vi "Video Toolset v10.0.0.vi"(9 "Capture Folder":path, 10 "Source Name":string, 11 "Autorun":bool) -> ()   [LabVIEW 2010]
uses:
  System.Windows.Forms
  drivers/DirectShow SDK/v10/DirectShow SDK.llb/DirectShow - Media State.ctl
  D:/Projekte/Promotion/Scripts/LabView/drivers/DirectShow SDK/lib/DirectShowLib-2005.dll
  drivers/DirectShow SDK/lib/DirectShowLib-2005.dll
  drivers/DirectShow SDK/v10/DirectShow SDK.llb/DirectShow - Capture Device.ctl
  drivers/DirectShow SDK/v10/DirectShow SDK.llb/DirectShow - Media Mode.ctl
  System.Drawing
  subvi/Remote Snapshot.vi
panel:
  in  "Autoclose":bool
  in  "Preview":refnum<k24>(container)
  in  "AutocloseText":string
  in  "AutorunText":string
  in  "Selector":u16(ring) items=["MJPG 1280x720, 30.00fps, 24bit", "MJPG 320x180, 30.00fps, 24bit", "MJPG 320x240, 30.00fps, 24bit", "MJPG 352x288, 30.00fps, 24bit", "MJPG 424x240, 30.00fps, 24bit", "MJPG 640x360, 30.00fps, 24bit", "MJPG 640x480, 30.00fps, 24bit", "MJPG 848x480, 30.00fps, 24bit", "MJPG 960x540, 30.00fps, 24bit", "YUY2 640x480, 30.00fps, 16bit", "YUY2 320x180, 30.00fps, 16bit", "YUY2 320x240, 30.00fps, 16bit", "YUY2 352x288, 30.00fps, 16bit", "YUY2 424x240, 30.00fps, 16bit", "YUY2 640x360, 30.00fps, 16bit", "YUY2 848x480, 20.00fps, 16bit", "YUY2 960x540, 15.00fps, 16bit", "YUY2 1280x720, 10.00fps, 16bit", "RGB 640x480, 30.00fps, 24bit", "RGB 320x180, 30.00fps, 24bit", "RGB 320x240, 30.00fps, 24bit", "RGB 352x288, 30.00fps, 24bit", "RGB 424x240, 30.00fps, 24bit", "RGB 640x360, 30.00fps, 24bit", "RGB 848x480, 20.00fps, 24bit", "RGB 960x540, 15.00fps, 24bit", "RGB 1280x720, 10.00fps, 24bit"]
  in  "WindowSnap":refnum<k24>(container)
  out "SnapSummary":string
  in  "Grab Window Image":bool
  in  "Pause":bool
  in  "Run":bool
  in  "Stop":bool
  in  "Capture":bool
  out "Summary":string
  in  "Grab Frame":bool
  in  "FrameGrab":refnum<k24>(container)
  out "Info":string
  in  "Fit Window":bool
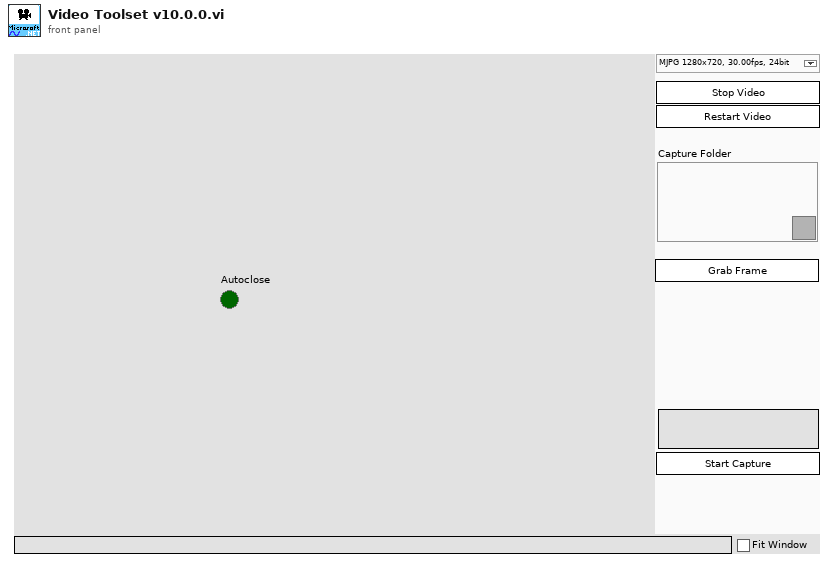
[diagram p1: front panel]
types:
  T1 = typedef "DirectShow - Media State.ctl" = enum16{"Stopped", "Playing", "Paused", "Recording"}
  T2 = typedef "DirectShow - Media Mode.ctl" = enum16{"Stop", "Run", "Pause"}
  T3 = typedef "DirectShow - Capture Device.ctl" = cluster{"DSDevice":refnum<k24>, "DevicePath":string, "Mon":refnum<k24>, "Name":string}
  T4 = enum8{"Enabled", "Disabled", "Disabled and Grayed Out"}
  T5 = enum16{"AnalogVideoIn", "Capture", "CC", "EDS", "NABTS", "Preview", "Still", "TeleText", "TimeCode", "VBI", "VideoPort", "VideoPortVBI"}
  T6 = cluster{"This VI":refnum<vi>, "Pane":refnum<vi>, "Timeout":i32, "Error":errorcluster, "Preview":refnum<k24>, "FrameGrab":refnum<k24>, "WindowSnap":refnum<k24>, "Video":T3, "Audio":T3, "VideoC":T3, "AudioC":T3, "Preview?":bool, "Capture?":bool, "ScaleWindow?":bool, "FrameGrabber?":bool, "IFilterGraph2":refnum<k24>, "ICaptureGraphBuilder2":refnum<k24>, "Video Caps":string[], "Audio Caps":string[], "CurrentVideo":string, "CurrentAudio":string, "MediaState":T1}
  T7 = typedef "sizeaction.ctl" = enum32{"Minimized", "Maximized", "Resized"}
  T8 = typedef "LVRectTypeDef.ctl" = cluster{"left":i16, "top":i16, "right":i16, "bottom":i16}
  T9 = cluster{"ID +Items":string[], "Items dup":string[], "Name":string}
  T10 = cluster{"ID +Items":string[], "Items dup":string[], "Name":string}[]
  T11 = typedef "imagedata.ctl" = cluster{"image type":i32, "image depth":i32, "image":u8[], "mask":u8[], "colors":u32[], "Rectangle":cluster{"left":i16, "top":i16, "right":i16, "bottom":i16}}
  T12 = enum32{"invalid app kind", "Development System", "Run Time System", "Student Edition", "Embedded LabVIEW", "Evaluation", "Custom"}
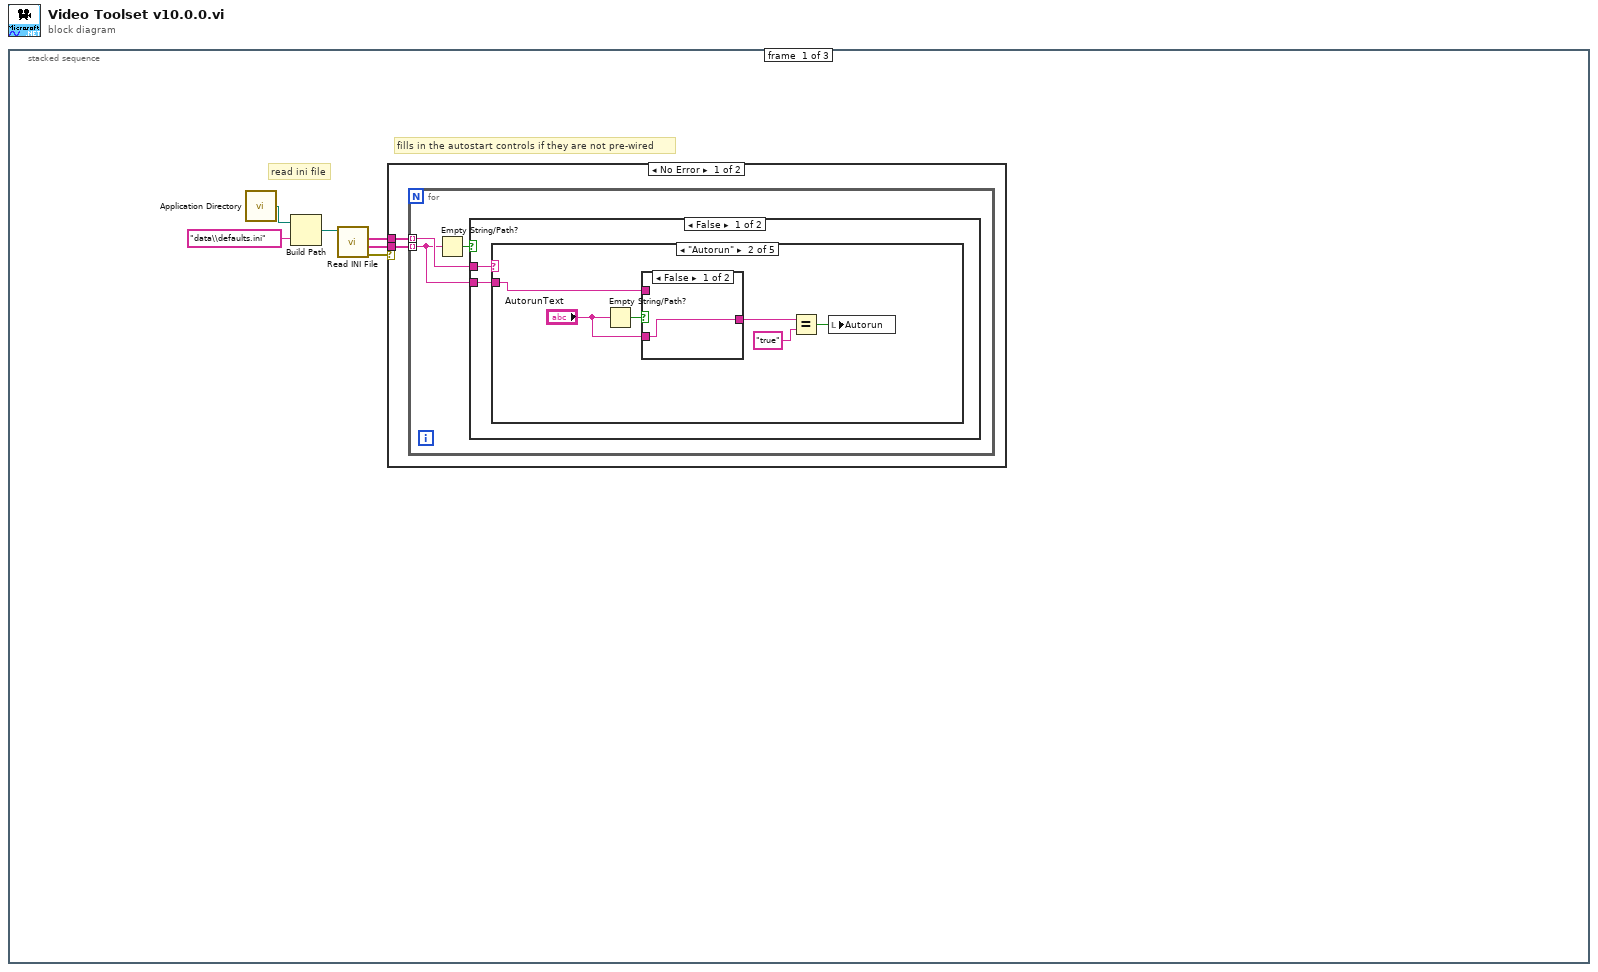
[diagram p0: block diagram]
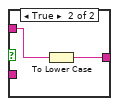
[diagram p3: hidden frame]
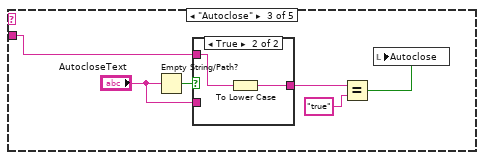
[diagram p4: hidden frame]
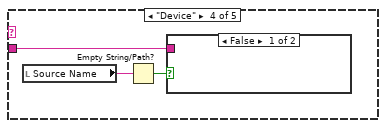
[diagram p6: hidden frame]
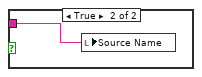
[diagram p7: hidden frame]
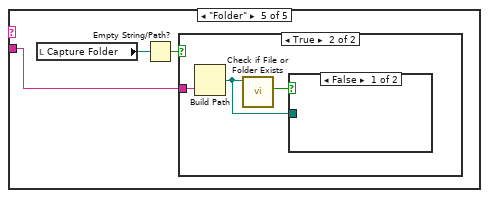
[diagram p8: hidden frame]
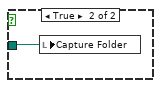
[diagram p10: hidden frame]
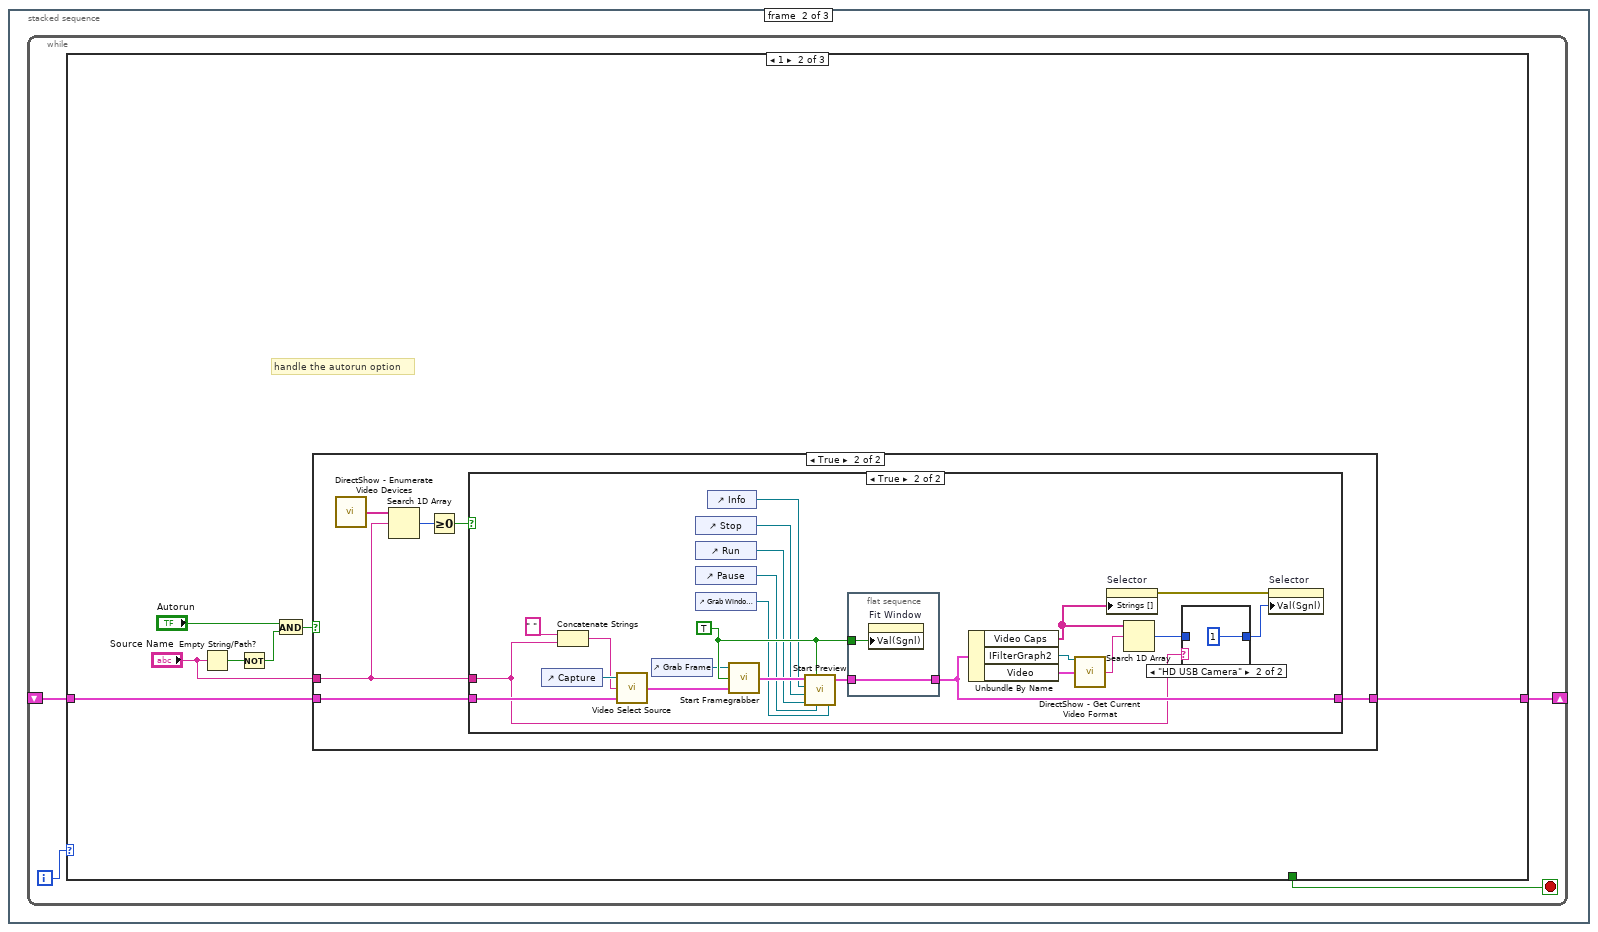
[diagram p13: hidden frame]
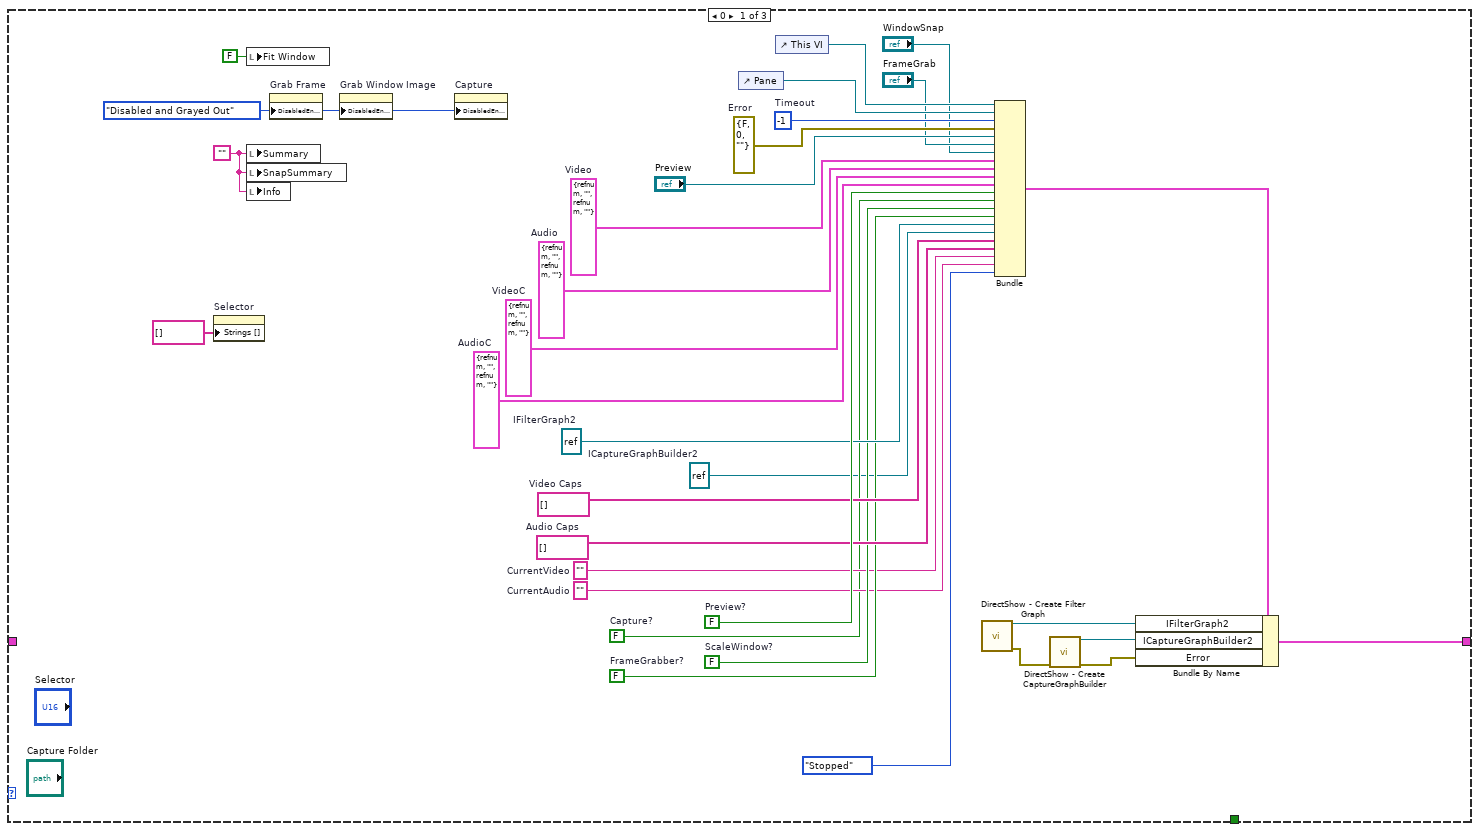
[diagram p14: hidden frame]
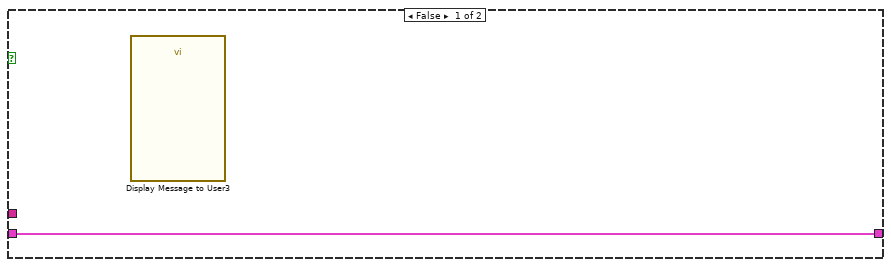
[diagram p16: hidden frame]
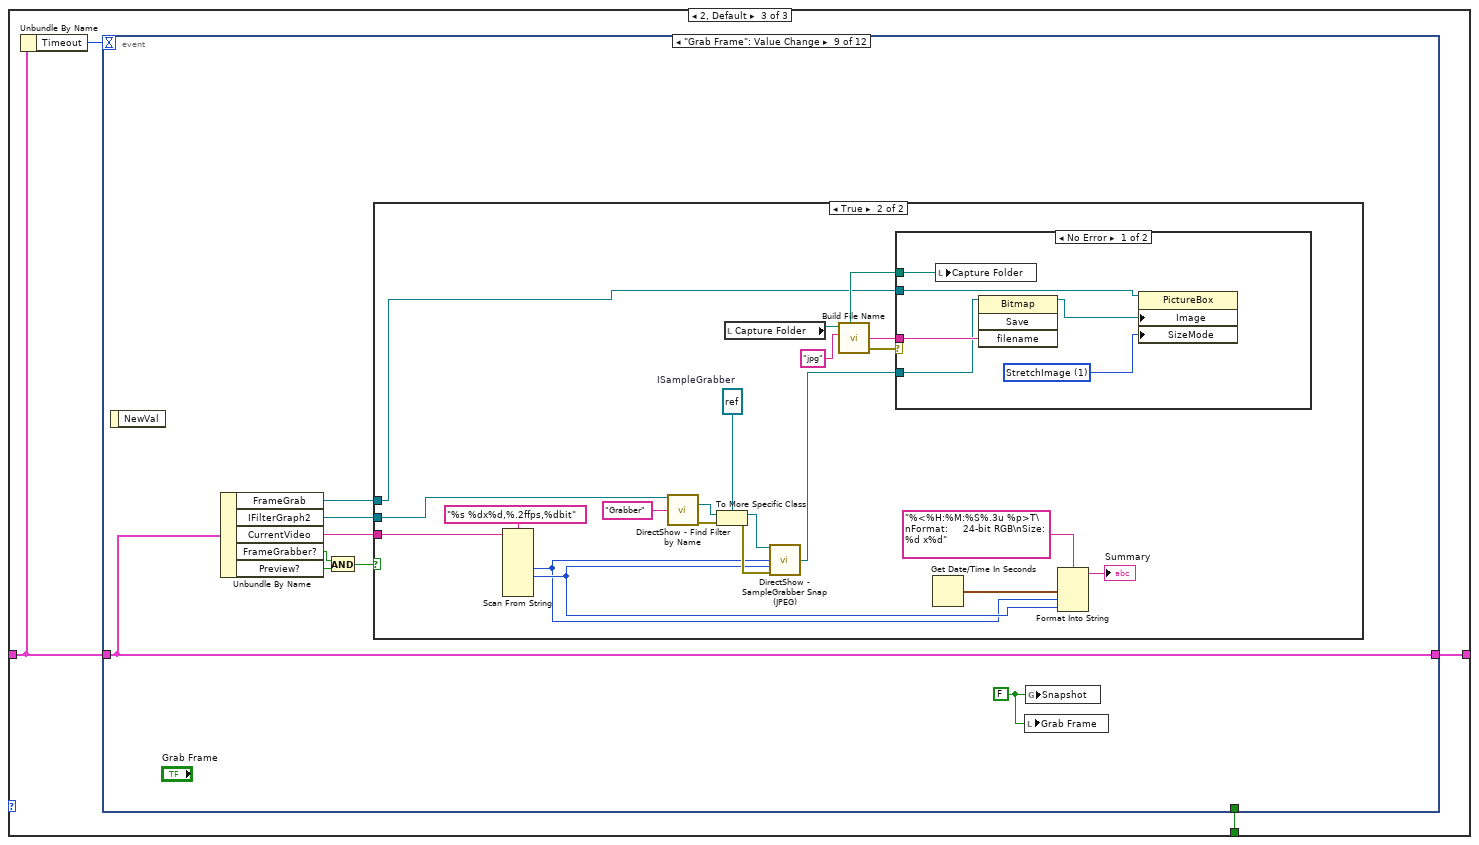
[diagram p18: hidden frame]
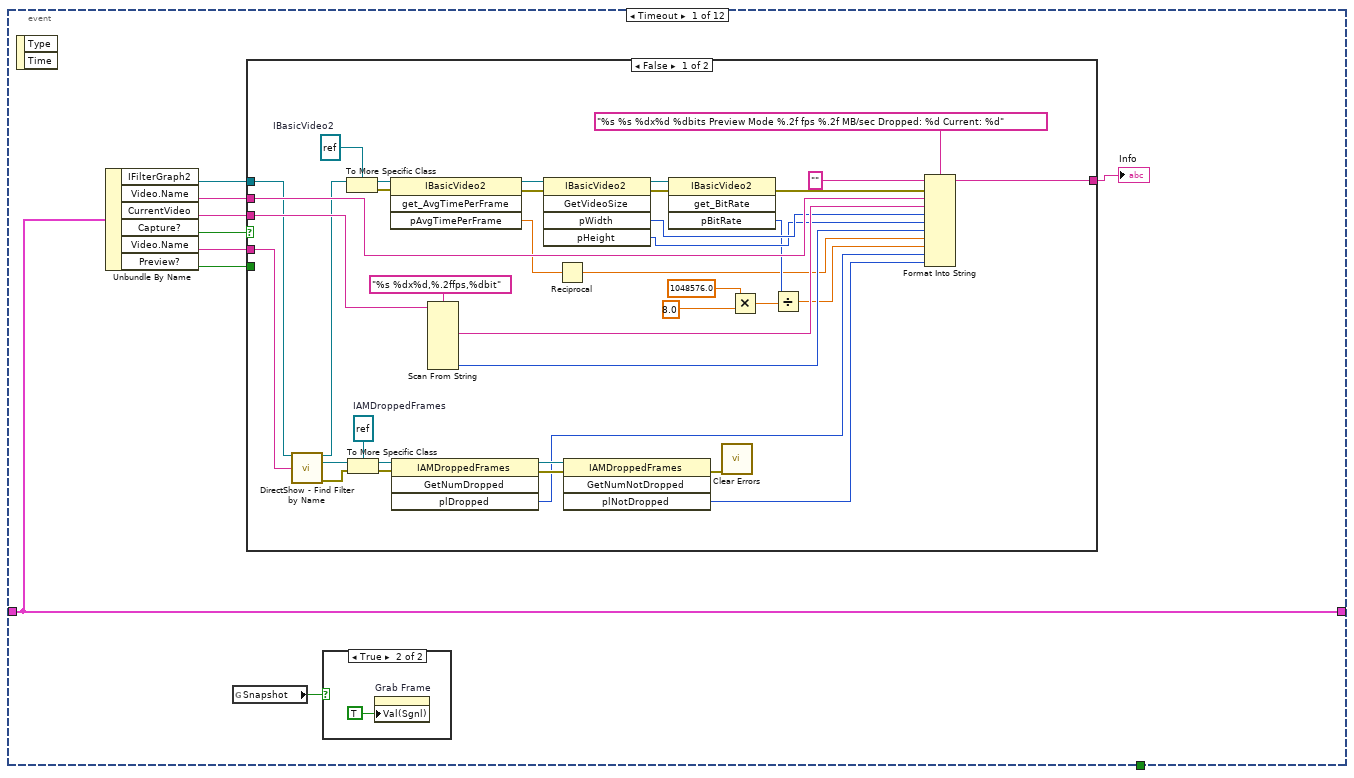
[diagram p19: hidden frame]
diagram:
  n1 = stacked-sequence {
    frame #0 {
      # "fills in the autostart controls if they are not pre-wired"
      # "read ini file"
      n2 = call <vilib>:"Application Directory.vi"() -> ("Application Directory"=w1:path)
      n3 = Build Path(base path=w1, name or relative path="data\\defaults.ini") -> (appended path=w5:path)
      n4 = call "Read INI File.vi"("configuration file path"=w5) -> ("error out"=w4:errorcluster, "values"=w2:string[], "keys"=w3:string[])  [unwired: 7 in, 1 out]
      n5 = case shown="No Error" w4 {
        tunnel: w3 -> [w8 _]
        tunnel: w2 -> [w7 _]
        frame No Error {
          n6 = for {
            tunnel: w8 -> [w10] mode=indexing
            tunnel: w7 -> [w9] mode=indexing
            n7 = Empty String/Path?(string/path=w9) -> (empty?=w11:bool)
            n8 = case shown="False" w11 {
              tunnel: w10 -> [w13 _]
              tunnel: w9 -> [w12 _]
              frame False {
                n9 = case shown="\"Autorun\"" w13 {
                  tunnel: w12 -> [_ w19 w23 w34 w38]
                  frame Default {
                  }
                  frame "Autorun" {
                    n10 = Empty String/Path?(string/path="AutorunText") -> (empty?=w17:bool)
                    n11 = case shown="False" w17 {
                      tunnel: w19 -> [_ w22]
                      tunnel: [w20 w21] -> w16
                      tunnel: "AutorunText" -> [w20 _]
                      frame False {
                      }
                      frame True {
                        n12 = To Lower Case(string=w22) -> (all lower case string=w21:string)
                      }
                    }
                    n13 = Equal?(x=w16, y="true") -> (x = y?=w14:bool)
                    n14 = local write "Autorun"(w14) -> ()
                  }
                  frame "Autoclose" {
                    n15 = Empty String/Path?(string/path="AutocloseText") -> (empty?=w24:bool)
                    n16 = case shown="True" w24 {
                      tunnel: [w29 w31] -> w27
                      tunnel: "AutocloseText" -> [w29 _]
                      tunnel: w23 -> [_ w30]
                      frame False {
                      }
                      frame True {
                        n17 = To Lower Case(string=w30) -> (all lower case string=w31:string)
                      }
                    }
                    n18 = Equal?(x=w27, y="true") -> (x = y?=w26:bool)
                    n19 = local write "Autoclose"(w26) -> ()
                  }
                  frame "Device" {
                    n20 = local read "Source Name"() -> (w33:string)
                    n21 = Empty String/Path?(string/path=w33) -> (empty?=w32:bool)
                    n22 = case shown="False" w32 {
                      tunnel: w34 -> [_ w35]
                      frame False {
                      }
                      frame True {
                        n23 = local write "Source Name"(w35) -> ()
                      }
                    }
                  }
                  frame "Folder" {
                    n24 = local read "Capture Folder"() -> (w37:path)
                    n25 = Empty String/Path?(string/path=w37) -> (empty?=w36:bool)
                    n26 = case shown="True" w36 {
                      tunnel: w38 -> [_ w41]
                      frame False {
                      }
                      frame True {
                        n27 = Build Path(name or relative path=w41) -> (appended path=w39:path)  [unwired: 1 in]
                        n28 = call <vilib>:"Check if File or Folder Exists.vi"("path"=w39) -> ("file or folder exists?"=w40:bool)  [unwired: 8 in, 2 out]
                        n29 = case shown="False" w40 {
                          tunnel: w39 -> [_ w42]
                          frame False {
                          }
                          frame True {
                            n30 = local write "Capture Folder"(w42) -> ()
                          }
                        }
                      }
                    }
                  }
                }
              }
              frame True {
              }
            }
          }
        }
        frame Error {
        }
      }
    }
    frame #1 {
      n31 = while {
        shift-right: [w45] -> _
        shift-left: _ -> [w44]
        i -> [w46]
        stop <- w43 stop-if-true
        n32 = case shown="1" w46 {
          tunnel: [w62 w81 w124] -> w45
          tunnel: w44 -> [_ w85 w123]
          tunnel: [_ _ w121] -> w43
          frame 0 {
            w47 = ""
            w55 = refnum<k24> refnum  # ICaptureGraphBuilder2
            w56 = FALSE  # Capture?
            w49 = T4."Disabled and Grayed Out" ("Disabled")
            w59 = ""  # CurrentAudio
            w60 = ""  # CurrentVideo
            w63 = FALSE  # FrameGrabber?
            w65 = FALSE  # ScaleWindow?
            w66 = string[] []  # Audio Caps
            w67 = string[] []  # Video Caps
            w70 = refnum<k24> refnum  # IFilterGraph2
            w71 = FALSE  # Preview?
            w72 = T3 {"DSDevice"=refnum, "DevicePath"="", "Mon"=refnum, "Name"=""}  # AudioC
            w73 = T3 {"DSDevice"=refnum, "DevicePath"="", "Mon"=refnum, "Name"=""}  # VideoC
            w74 = T3 {"DSDevice"=refnum, "DevicePath"="", "Mon"=refnum, "Name"=""}  # Audio
            w75 = T3 {"DSDevice"=refnum, "DevicePath"="", "Mon"=refnum, "Name"=""}  # Video
            w77 = errorcluster {"status"=FALSE, "code"=0, "source"=""}  # Error
            w78 = -1  # Timeout
            n33 = property on="Selector" class="Ring (strict)"("Strings []"=string[] []) -> ()  [unwired: 2 in, 2 out]
            n34 = local write "Fit Window"(FALSE ("Fit Window")) -> ()
            n35 = local write "Summary"(w47) -> ()
            n36 = local write "SnapSummary"(w47) -> ()
            n37 = local write "Info"(w47) -> ()
            n38 = property on="Grab Frame" class="Bool (strict)"("DisabledEnum"=w49) -> ()  [unwired: 2 in, 2 out]
            n39 = property on="Grab Window Image" class="Bool"("DisabledEnum"=w49) -> ()  [unwired: 2 in, 2 out]
            n40 = property on="Capture" class="Bool (strict)"("DisabledEnum"=w49) -> ()  [unwired: 2 in, 2 out]
            n41 = control-ref of="Pane"() -> (w58:refnum<vi>)
            n42 = control-ref of="This VI"() -> (w64:refnum<vi>)
            n43 = call "DirectShow - Create Filter Graph.vi"() -> ("IFilterGraph2"=w61:refnum<k24>, "error out"=w53:errorcluster)  [unwired: 14 in]
            n44 = Bundle("This VI"=w64, "Pane"=w58, "Timeout"=w78, "Error"=w77, "Preview"="Preview", "FrameGrab"="FrameGrab", "WindowSnap"="WindowSnap", "Video"=w75, "Audio"=w74, "VideoC"=w73, "AudioC"=w72, "Preview?"=w71, "Capture?"=w56, "ScaleWindow?"=w65, "FrameGrabber?"=w63, "IFilterGraph2"=w70, "ICaptureGraphBuilder2"=w55, "Video Caps"=w67, "Audio Caps"=w66, "CurrentVideo"=w60, "CurrentAudio"=w59, "MediaState"=DirectShow_-_Media_State."Stopped") -> (w68:T6)  [unwired: 1 in]
            n45 = call "DirectShow - Create CaptureGraphBuilder.vi"("error in (no error)"=w53) -> ("ICaptureGraphBuilder2"=w54:refnum<k24>, "error out"=w52:errorcluster)  [unwired: 13 in]
            n46 = Bundle By Name(cluster=w68, "IFilterGraph2"=w61, "ICaptureGraphBuilder2"=w54, "Error"=w52) -> (w62:T6)
          }
          frame 1 {
            # "handle the autorun option"
            n47 = Empty String/Path?(string/path="Source Name") -> (empty?=w80:bool)
            n48 = Not(x=w80) -> (.not. x?=w79:bool)
            n49 = And(x="Autorun", y=w79) -> (x .and. y?=w82:bool)
            n50 = case shown="True" w82 {
              tunnel: w85 -> [w86 w92]
              tunnel: "Source Name" -> [_ w90]
              tunnel: [w86 w91] -> w81
              frame False {
              }
              frame True {
                n51 = call "DirectShow - Enumerate Video Devices.vi"() -> ("Names"=w89:string[])  [unwired: 13 in, 2 out]
                n52 = Search 1D Array(1D array=w89, element=w90) -> (index of element=w88:i32)  [unwired: 1 in]
                n53 = Greater Or Equal To 0?(x=w88) -> (x >= 0?=w87:bool)
                n54 = case shown="True" w87 {
                  tunnel: w92 -> [w93 w115]
                  tunnel: [w93 w101] -> w91
                  tunnel: w90 -> [_ w97]
                  frame False {
                    n55 = call "Display Message to User3"() -> ()  [unwired: 10 in, 2 out]
                  }
                  frame True {
                    w116 = TRUE ("Value (Signaling)")
                    n56 = control-ref of="Capture"() -> (w112:refnum<vi>)
                    n57 = Concatenate Strings(" " ("string"), w97) -> (w104:string)
                    n58 = call "Video Select Source.vi"("Cluster In"=w115, "Source Name"=w104, "Bool Refnum"=w112) -> ("Cluster Out"=w114:T6)
                    n59 = control-ref of="Grab Frame"() -> (w111:refnum<vi>)
                    n60 = control-ref of="Stop"() -> (w106:refnum<vi>)
                    n61 = control-ref of="Run"() -> (w108:refnum<vi>)
                    n62 = control-ref of="Pause"() -> (w109:refnum<vi>)
                    n63 = control-ref of="Grab Window Image"() -> (w110:refnum<vi>)
                    n64 = control-ref of="Info"() -> (w107:refnum<vi>)
                    n65 = call "Start Framegrabber.vi"("Cluster In"=w114, "Enable?"=w116, "Bool Refnum"=w111) -> ("Cluster Out"=w113:T6)
                    n66 = call "Start Preview.vi"("Cluster In"=w113, "Start?"=w116, "Info"=w107, "Stop"=w106, "Pause"=w109, "Run"=w108, "Grab Window Image"=w110) -> ("Cluster Out"=w103:T6)  [unwired: 1 in]
                    n67 = flat-sequence {
                      tunnel: w116 -> [w120]
                      tunnel: [w119] -> w101
                      tunnel: w103 -> [w119]
                      frame #0 {
                        n68 = property on="Fit Window" class="Bool (strict)"("Val(Sgnl)"=w120) -> ()  [unwired: 2 in, 2 out]
                      }
                    }
                    n69 = Unbundle By Name(w101) -> ("Video Caps"=w102:string[], "IFilterGraph2"=w98:refnum<k24>, "Video"=w99:T3)
                    n70 = call "DirectShow - Get Current Video Format.vi"("IFilterGraph2"=w98, "Video"=w99) -> ("Abbreviated"=w100:string)  [unwired: 10 in, 3 out]
                    n71 = property on="Selector" class="Ring (strict)"("Strings []"=w102) -> (error out=w96:errorcluster)  [unwired: 2 in, 1 out]
                    n72 = Search 1D Array(1D array=w102, element=w100) -> (index of element=w94:i32)  [unwired: 1 in]
                    n73 = case shown="\"HD USB Camera\"" w97 {
                      tunnel: [w117 u16 1 ("Value (Signaling)")] -> w95
                      tunnel: w94 -> [w117 _]
                      frame "False", Default {
                      }
                      frame "HD USB Camera" {
                      }
                    }
                    n74 = property on="Selector" class="Ring (strict)"(error in=w96, "Val(Sgnl)"=w95) -> ()  [unwired: 1 in, 2 out]
                  }
                }
              }
            }
          }
          frame 2, Default {
            n75 = Unbundle By Name(w123) -> ("Timeout"=w122:i32)
            n76 = event shown="[8] \"Grab Frame\": Value Change" {
              selector: _ -> [_ _ _ _ _ _ _ _ _ _ _ _]
              dyn-events: _ -> [_ _ _ _ _ _ _ _ _ _ _ _]
              timeout: w122 -> [_ _ _ _ _ _ _ _ _ _ _ _]
              tunnel: [w133 w204 w226 w285 w395 w999 w1078 w1102 w1126 w1160 w1183 w1318] -> w124
              tunnel: w123 -> [w133 w204 w227 w306 w394 w1000 w1077 w1101 w1126 w1160 w1182 w1318]
              tunnel: [_ w208 _ _ w393 _ _ _ _ _ _ _] -> w121
              event Timeout {
                n77 = event-data() -> ()  [unwired: 1 in, 2 out]
                n78 = Unbundle By Name(w133) -> ("IFilterGraph2"=w132:refnum<k24>, "Video.Name"=w130:string, "CurrentVideo"=w131:string, "Capture?"=w129:bool, "Video.Name"=w127:string, "Preview?"=w126:bool)
                n79 = global read "Remote Snapshot.vi" "Snapshot"() -> (w125:bool)
                n80 = case shown="False" w129 {
                  tunnel: w132 -> [w144 w187]
                  tunnel: w131 -> [w162 w182]
                  tunnel: w130 -> [w160 w184]
                  tunnel: [w150 w185] -> w128
                  tunnel: w127 -> [w145 w188]
                  tunnel: w126 -> [_ _]
                  frame False {
                    w149 = refnum<k24> refnum  # IAMDroppedFrames
                    w172 = refnum<k24> refnum  # IBasicVideo2
                    n81 = call "DirectShow - Find Filter by Name.vi"("IFilterGraph2"=w144, "pName"=w145) -> ("IFilterGraph2 dup"=w143:refnum<k24>, "ppFilter"=w148:refnum<k24>, "error out"=w142:errorcluster)  [unwired: 11 in]
                    n82 = To More Specific Class(target class=w172, reference=w143) -> (specific class reference=w171:refnum<k24>, error out=w170:errorcluster)  [unwired: 1 in]
                    n83 = To More Specific Class(target class=w149, reference=w148, error in=w142) -> (specific class reference=w139:refnum<k24>, error out=w138:errorcluster)
                    n84 = invoke class="IBasicVideo2" method="get_AvgTimePerFrame"(reference=w171, error in=w170) -> (reference out=w169:refnum<k24>, error out=w168:errorcluster, "pAvgTimePerFrame"=w152:dbl)  [unwired: 2 in, 1 out]
                    n85 = invoke class="IAMDroppedFrames" method="GetNumDropped"(reference=w139, error in=w138) -> (reference out=w147:refnum<k24>, error out=w146:errorcluster, "plDropped"=w137:i32)  [unwired: 2 in, 1 out]
                    n86 = Scan From String(format string="%s %dx%d,%.2ffps,%dbit", input string=w162) -> (output 1=w159:string, output 5=w158:i32)  [unwired: 10 in, 3 out]
                    n87 = invoke class="IBasicVideo2" method="GetVideoSize"(reference=w169, error in=w168) -> (reference out=w167:refnum<k24>, error out=w166:errorcluster, "pWidth"=w157:i32, "pHeight"=w156:i32)  [unwired: 3 in, 1 out]
                    n88 = Reciprocal(x=w152) -> (1/x=w151:dbl)
                    n89 = invoke class="IAMDroppedFrames" method="GetNumNotDropped"(reference=w147, error in=w146) -> (error out=w135:errorcluster, "plNotDropped"=w136:i32)  [unwired: 2 in, 2 out]
                    n90 = invoke class="IBasicVideo2" method="get_BitRate"(reference=w167, error in=w166) -> (error out=w165:errorcluster, "pBitRate"=w155:i32)  [unwired: 2 in, 2 out]
                    n91 = call <vilib>:"Clear Errors.vi"("error in (no error)"=w135) -> ()  [unwired: 6 in, 1 out]
                    n92 = Multiply(x=1048576.0, y=8.0) -> (x*y=w141:dbl)
                    n93 = Divide(x=w155, y=w141) -> (x/y=w153:dbl)
                    n94 = Format Into String(format string="%s %s %dx%d %dbits Preview Mode %.2f fps %.2f MB/sec Dropped: %d Current: %d", initial string="", error in=w165, w160, w159, w157, w156, w158, w151, w153, w137, w136) -> (resulting string=w150:string)  [unwired: 1 out]
                  }
                  frame True {
                    w192 = refnum<k24> refnum  # IAMDroppedFrames
                    n95 = call "DirectShow - Find Filter by Name.vi"("IFilterGraph2"=w187, "pName"=w188) -> ("ppFilter"=w191:refnum<k24>, "error out"=w190:errorcluster)  [unwired: 11 in, 1 out]
                    n96 = To More Specific Class(target class=w192, reference=w191, error in=w190) -> (specific class reference=w173:refnum<k24>, error out=w189:errorcluster)
                    n97 = Scan From String(format string="%s %dx%d,%.2ffps,%dbit", input string=w182) -> (output 1=w181:string, output 2=w180:i32, output 3=w179:i32, output 4=w177:dbl, output 5=w178:i32)  [unwired: 7 in, 3 out]
                    n98 = Not A Number/Path/Refnum?(number/path/refnum=w173) -> (NaN/Path/Refnum?=w174:bool)
                    n99 = case shown="False" w174 {
                      tunnel: w173 -> [w196 _]
                      tunnel: w189 -> [w195 _]
                      tunnel: [w194 w199] -> w176
                      tunnel: [w193 w199] -> w175
                      frame False {
                        n100 = invoke class="IAMDroppedFrames" method="GetNumDropped"(reference=w196, error in=w195) -> (reference out=w198:refnum<k24>, error out=w197:errorcluster, "plDropped"=w194:i32)  [unwired: 2 in, 1 out]
                        n101 = invoke class="IAMDroppedFrames" method="GetNumNotDropped"(reference=w198, error in=w197) -> ("plNotDropped"=w193:i32)  [unwired: 2 in, 3 out]
                      }
                      frame True {
                        w199 = 0 ("plDropped")
                      }
                    }
                    n102 = Format Into String(format string="%s %s %dx%d %dbits Capture Mode %.2f fps Dropped: %d Current: %d", w184, w181, w180, w179, w178, w177, w176, w175) -> (resulting string=w185:string)  [unwired: 2 in, 1 out]
                  }
                }
                "Info" <- w128
                n103 = case shown="True" w125 {
                  frame False {
                  }
                  frame True {
                    n104 = property on="Grab Frame" class="Bool (strict)"("Val(Sgnl)"=TRUE) -> ()  [unwired: 2 in, 2 out]
                  }
                }
              }
              event Panel Close? {
                w208 = TRUE ("Discard?")
                n105 = event-data() -> ()  [unwired: 1 in, 3 out]
                n106 = Unbundle By Name(w204) -> ("ICaptureGraphBuilder2"=w200:refnum<k24>, "Capture?"=w201:bool, "IFilterGraph2"=w207:refnum<k24>, "Error"=w206:errorcluster, "Preview?"=w205:bool)
                n107 = case shown="True" w205 {
                  tunnel: w207 -> [w210 w218]
                  tunnel: w206 -> [w209 _]
                  tunnel: [w210 w213] -> w203
                  tunnel: [w209 w211] -> w202
                  tunnel: w201 -> [_ w216]
                  tunnel: w200 -> [_ w215]
                  frame False {
                  }
                  frame True {
                    n108 = call "DirectShow - Media Control - StartStopPause.vi"("IFilterGraph2"=w218, "Mode"=DirectShow_-_Media_Mode."Stop") -> ("IFilterGraph2 dup"=w212:refnum<k24>, "error out"=w214:errorcluster)  [unwired: 12 in]
                    n109 = case shown="True" w216 {
                      tunnel: w215 -> [_ w224]
                      tunnel: w214 -> [w219 w223]
                      tunnel: [w220 w222] -> w213
                      tunnel: w212 -> [w220 w222]
                      tunnel: [w219 w221] -> w211
                      frame False {
                      }
                      frame True {
                        n110 = call "DirectShow - Release Object.vi"("o"=w224, "error in (no error)"=w223) -> ("error out"=w221:errorcluster)  [unwired: 13 in]
                      }
                    }
                  }
                }
                n111 = call "DirectShow - Release Object.vi"("o"=w203, "error in (no error)"=w202) -> ()  [unwired: 13 in, 1 out]
                n112 = event-data("Discard?"=w208) -> ()  [unwired: 1 in, 1 out]
              }
              event Panel Resize {
                n113 = event-data() -> ("Act"=w225:T7)  [unwired: 1 in]
                n114 = case shown="\"Maximized\", Default" w225 {
                  tunnel: w227 -> [w228 w235]
                  tunnel: [w228 w234] -> w226
                  frame "Minimized" {
                  }
                  frame "Maximized", Default {
                    n115 = Unbundle By Name(w235) -> ("Pane"=w232:refnum<vi>, "Error"=w233:errorcluster, "IFilterGraph2"=w231:refnum<k24>, "ScaleWindow?"=w229:bool)
                    n116 = case shown="True" w229 {
                      tunnel: w233 -> [w236 w247]
                      tunnel: w232 -> [_ w246]
                      tunnel: w231 -> [_ w244]
                      tunnel: [w236 w240] -> w230
                      frame False {
                      }
                      frame True {
                        w239 = 0 ("left")
                        w245 = refnum<k24> refnum  # IVideoWindow
                        n117 = property class="Pane"(reference=w246, error in=w247) -> (error out=w243:errorcluster, "ContentBnds"=w252:T8)  [unwired: 1 out]
                        n118 = Unbundle(w252) -> ("left"=w248:i16, "top"=w250:i16, "right"=w249:i16, "bottom"=w251:i16)
                        n119 = Subtract(x=w249, y=w248) -> (x-y=w238:i16)
                        n120 = Subtract(x=w251, y=w250) -> (x-y=w237:i16)
                        n121 = To More Specific Class(target class=w245, reference=w244, error in=w243) -> (specific class reference=w242:refnum<k24>, error out=w241:errorcluster)
                        n122 = invoke class="IVideoWindow" method="SetWindowPosition"(reference=w242, error in=w241, "left"=w239, "top"=w239, "width"=w238, "height"=w237) -> (error out=w240:errorcluster)  [unwired: 1 in, 6 out]
                      }
                    }
                    n123 = Bundle By Name(cluster=w235, "Error"=w230) -> (w234:T6)
                  }
                }
              }
              event Menu Activation? {
                w271 = "(none)" ("Name")
                # "Disable Menu When in Capture Mode"
                n124 = event-data() -> ("MenuRef"=w257:refnum<k9>)  [unwired: 1 in]
                n125 = call "DirectShow - Enumerate Video Devices.vi"() -> ("Names"=w323:string[])  [unwired: 13 in, 2 out]
                n126 = call "DirectShow - Enumerate Audio Devices.vi"() -> ("Names"=w322:string[])  [unwired: 13 in, 2 out]
                n127 = call "DirectShow - Enumerate Video Compressors.vi"() -> ("Names"=w321:string[])  [unwired: 13 in, 2 out]
                n128 = call "DirectShow - Enumerate Audio Compressors.vi"() -> ("Names"=w320:string[])  [unwired: 13 in, 2 out]
                n129 = call "Logical String Array Sort.vi"("Unsorted List"=w323) -> ("Sorted List"=w298:string[])  [unwired: 18 in]
                n130 = call "Logical String Array Sort.vi"("Unsorted List"=w322) -> ("Sorted List"=w297:string[])  [unwired: 18 in]
                n131 = call "Logical String Array Sort.vi"("Unsorted List"=w321) -> ("Sorted List"=w296:string[])  [unwired: 18 in]
                n132 = call "Logical String Array Sort.vi"("Unsorted List"=w320) -> ("Sorted List"=w295:string[])  [unwired: 18 in]
                n133 = Build Array (concatenate)(w271, w298) -> (w277:string[])
                n134 = Build Array (concatenate)(w271, w297) -> (w273:string[])
                n135 = Build Array (concatenate)(w271, w296) -> (w270:string[])
                n136 = Build Array (concatenate)(w271, w295) -> (w269:string[])
                n137 = Unbundle By Name(w306) -> ("Capture?"=w258:bool, "Preview?"=w259:bool, "Video.Name"=w289:string, "Audio.Name"=w290:string, "VideoC.Name"=w309:string, "AudioC.Name"=w319:string)
                n138 = call "DirectShow - Menu - Append Item ID.vi"("ID"="Video:" ("tag"), "Items"=w277) -> ("ID +Items"=w274:string[], "Items dup"=w275:string[])  [unwired: 12 in]
                n139 = call "DirectShow - Menu - Append Item ID.vi"("ID"="VideoC:" ("tag"), "Items"=w270) -> ("ID +Items"=w265:string[], "Items dup"=w262:string[])  [unwired: 12 in]
                n140 = call "DirectShow - Menu - Append Item ID.vi"("ID"="Audio:" ("tag"), "Items"=w273) -> ("ID +Items"=w266:string[], "Items dup"=w263:string[])  [unwired: 12 in]
                n141 = call "DirectShow - Menu - Append Item ID.vi"("ID"="AudioC:" ("tag"), "Items"=w269) -> ("ID +Items"=w264:string[], "Items dup"=w261:string[])  [unwired: 12 in]
                n142 = Not(x=w258) -> (.not. x?=w253:bool)
                n143 = Bundle("ID +Items"=w274, "Items dup"=w275, "Name"=w289) -> (w328:T9)  [unwired: 1 in]
                n144 = Bundle("ID +Items"=w266, "Items dup"=w263, "Name"=w290) -> (w327:T9)  [unwired: 1 in]
                n145 = Bundle("ID +Items"=w265, "Items dup"=w262, "Name"=w309) -> (w326:T9)  [unwired: 1 in]
                n146 = Bundle("ID +Items"=w264, "Items dup"=w261, "Name"=w319) -> (w325:T9)  [unwired: 1 in]
                n147 = Build Array(w328, w327, w326, w325) -> (w324:T10)
                n148 = Not(x=w259) -> (.not. x?=w260:bool)
                n149 = for {
                  tunnel: w257 -> [w345]
                  tunnel: string[] ["Video Devices", "Audio Devices", "Video Compressors", "Audio Compressors"] -> [w344] mode=indexing
                  tunnel: w324 -> [w343] mode=indexing
                  tunnel: [w338] -> w318
                  tunnel: [w337] -> w317
                  tunnel: w260 -> [w336]
                  n150 = Unbundle(w343) -> ("ID +Items"=w341:string[], "Items dup"=w342:string[], "Name"=w339:string)
                  n151 = Empty String/Path?(string/path=w339) -> (empty?=w340:bool)
                  n152 = case shown="True" w340 {
                    tunnel: w345 -> [w359 w382]
                    tunnel: w344 -> [w351 w374]
                    tunnel: w342 -> [w348 w369]
                    tunnel: w341 -> [w347 w370]
                    tunnel: w339 -> [_ w373]
                    tunnel: [w350 w372] -> w338
                    tunnel: [w349 w371] -> w337
                    tunnel: w336 -> [w346 w368]
                    frame True {
                      n153 = Get Menu Item Info(7:w351, 11:w359) -> (0:w356:errorcluster, 3:w357:refnum<k9>, 5:w358:string[])  [unwired: 1 in, 4 out]
                      n154 = Delete Menu Items(6:w356, 7:w358, 8:w351, 9:w357) -> (0:w354:errorcluster, 3:w355:refnum<k9>)
                      n155 = Insert Menu Items(5:w351, 6:w354, 7:w347, 8:w348, 9:w355) -> (0:w353:errorcluster, 3:w352:refnum<k9>)  [unwired: 1 in, 1 out]
                      n156 = for {
                        shift-right: [w365] -> w350
                        shift-left: w352 -> [w366]
                        shift-right: [w364] -> w349
                        shift-left: w353 -> [w367]
                        tunnel: w347 -> [w363] mode=indexing
                        tunnel: w346 -> [w360]
                        i -> [w361]
                        n157 = Equal To 0?(x=w361) -> (x = 0?=w362:bool)
                        n158 = Set Menu Item Info(6:w362, 7:w363, 8:w367, 9:w360, 11:w366) -> (0:w364:errorcluster, 3:w365:refnum<k9>)  [unwired: 2 in]
                      }
                    }
                    frame False {
                      n159 = Get Menu Item Info(7:w374, 11:w382) -> (0:w379:errorcluster, 3:w380:refnum<k9>, 5:w381:string[])  [unwired: 1 in, 4 out]
                      n160 = Delete Menu Items(6:w379, 7:w381, 8:w374, 9:w380) -> (0:w377:errorcluster, 3:w378:refnum<k9>)
                      n161 = Insert Menu Items(5:w374, 6:w377, 7:w370, 8:w369, 9:w378) -> (0:w376:errorcluster, 3:w375:refnum<k9>)  [unwired: 1 in, 1 out]
                      n162 = for {
                        shift-right: [w389] -> w372
                        shift-left: w375 -> [w390]
                        shift-right: [w388] -> w371
                        shift-left: w376 -> [w391]
                        tunnel: w370 -> [w387] mode=indexing
                        tunnel: w373 -> [w385]
                        tunnel: w369 -> [w386] mode=indexing
                        tunnel: w368 -> [w383]
                        n163 = Equal?(x=w386, y=w385) -> (x = y?=w384:bool)
                        n164 = Set Menu Item Info(6:w384, 7:w387, 8:w391, 9:w383, 11:w390) -> (0:w388:errorcluster, 3:w389:refnum<k9>)  [unwired: 2 in]
                      }
                    }
                  }
                }
                n165 = Empty String/Path?(string/path=w289) -> (empty?=w313:bool)
                n166 = Empty String/Path?(string/path=w290) -> (empty?=w312:bool)
                n167 = Not(x=w313) -> (.not. x?=w256:bool)
                n168 = Not(x=w312) -> (.not. x?=w280:bool)
                n169 = Unbundle By Name(w306) -> ("Video Caps"=w303:string[], "Audio Caps"=w300:string[], "FrameGrabber?"=w291:bool, "IFilterGraph2"=w288:refnum<k24>, "Video"=w279:T3, "Audio"=w278:T3)
                n170 = Empty String/Path?(string/path=w309) -> (empty?=w307:bool)
                n171 = Not(x=w307) -> (.not. x?=w308:bool)
                n172 = Unbundle By Name(w306) -> ("Preview?"=w254:bool)
                n173 = And(x=w254, y=w280) -> (x .and. y?=w281:bool)
                n174 = And(x=w254, y=w256) -> (x .and. y?=w282:bool)
                n175 = Or(x=w256, y=w280) -> (x .or. y?=w310:bool)
                n176 = Build Array(w256, w280, w310, w256, w256, w308, w280, w256, w256, w256, w256, w280, w280, w280, w256, w280, w282, w281, w253, w253) -> (w311:bool[])
                n177 = for {
                  tunnel: w318 -> [w335]
                  tunnel: w317 -> [w334]
                  tunnel: string[] ["Video Compressors", "Audio Compressors", "Property Pages", "Video Capture Device", "Video Capture Pin", "Video Compressor", "Audio Capture Device", "Video Frame Format", "Video Frame Bits", "Video Frame Size", "Video Frame Rate", "Audio Channels", "Audio Sampling Rate", "Audio Sample Size", "Video Capabilities", "Audio Capabilities", "Video Renderer Stats", "Audio Renderer Stats", "Devices", "Options"] -> [w333] mode=indexing
                  tunnel: [w332] -> w315
                  tunnel: [w331] -> w314
                  tunnel: w311 -> [w330] mode=indexing
                  n178 = Set Menu Item Info(7:w333, 8:w334, 9:w330, 11:w335) -> (0:w331:errorcluster, 3:w332:refnum<k9>)  [unwired: 3 in]
                }
                n179 = call "DirectShow - Get Current Video Format.vi"("IFilterGraph2"=w288, "Video"=w279) -> ("IFIlterGraph2 dup"=w286:refnum<k24>, "Abbreviated"=w284:string, "error out"=w287:errorcluster)  [unwired: 10 in, 1 out]
                n180 = Set Menu Item Info(6:w254, 7:"Preview", 8:w314, 9:w256, 11:w315) -> (0:w304:errorcluster, 3:w305:refnum<k9>)  [unwired: 2 in]
                n181 = call "DirectShow - Get Current Audio Format.vi"("IFilterGraph2"=w286, "Audio"=w278, "error in (no error)"=w287) -> ("Abbreviated"=w283:string)  [unwired: 9 in, 3 out]
                n182 = call "DirectShow - Menu - Add Video Items.vi"("Menu"=w305, "Video Caps"=w303, "CurrentVideo"=w284, "error in (no error)"=w304) -> ("Menu out"=w302:refnum<k9>, "error out"=w301:errorcluster)  [unwired: 10 in]
                n183 = call "DirectShow - Menu - Add Audio Items.vi"("Menu"=w302, "Audio Caps"=w300, "CurrentAudio"=w283, "error in (no error)"=w301) -> ("Menu out"=w294:refnum<k9>, "error out"=w293:errorcluster)  [unwired: 10 in]
                n184 = Bundle By Name(cluster=w306, "CurrentVideo"=w284, "CurrentAudio"=w283) -> (w285:T6)
                n185 = Compound Arithmetic op=AND(w256, w253, invert w254) -> (w255:bool)
                n186 = Set Menu Item Info(6:w291, 7:"Enable Frame Grabber", 8:w293, 9:w255, 11:w294) -> ()  [unwired: 2 in, 2 out]
                n187 = event-data() -> ()  [unwired: 2 in, 1 out]
              }
              event Menu Selection (User) {
                n188 = event-data() -> ("MenuRef"=w392:refnum<k9>, "ItemTag"=w396:string)  [unwired: 1 in]
                n189 = case shown="\"Unknown\", Default" w396 {
                  selector: w396 -> [_ w431 w928 w935 _ _ _ _]
                  tunnel: [w399 w422 w919 w936 w945 w950 w972 w994] -> w395
                  tunnel: w394 -> [w399 w428 w920 w932 w945 w950 w972 w994]
                  tunnel: [TRUE _ _ _ _ _ _ _] -> w393
                  tunnel: w392 -> [_ _ w931 w940 _ _ _ _]
                  frame "Exit" {
                    n190 = Unbundle By Name(w399) -> ("ICaptureGraphBuilder2"=w398:refnum<k24>, "Capture?"=w397:bool, "IFilterGraph2"=w404:refnum<k24>, "Error"=w403:errorcluster, "Preview?"=w402:bool)
                    n191 = case shown="True" w402 {
                      tunnel: w404 -> [w407 w415]
                      tunnel: w403 -> [w406 _]
                      tunnel: [w407 w412] -> w401
                      tunnel: [w406 w411] -> w400
                      tunnel: w398 -> [_ w409]
                      tunnel: w397 -> [_ w408]
                      frame False {
                      }
                      frame True {
                        n192 = call "DirectShow - Media Control - StartStopPause.vi"("IFilterGraph2"=w415, "Mode"=DirectShow_-_Media_Mode."Stop") -> ("IFilterGraph2 dup"=w410:refnum<k24>, "error out"=w413:errorcluster)  [unwired: 12 in]
                        n193 = case shown="True" w408 {
                          tunnel: w409 -> [_ w421]
                          tunnel: w413 -> [w416 w420]
                          tunnel: [w417 w419] -> w412
                          tunnel: w410 -> [w417 w419]
                          tunnel: [w416 w418] -> w411
                          frame False {
                          }
                          frame True {
                            n194 = call "DirectShow - Release Object.vi"("o"=w421, "error in (no error)"=w420) -> ("error out"=w418:errorcluster)  [unwired: 13 in]
                          }
                        }
                      }
                    }
                    n195 = call "DirectShow - Release Object.vi"("o"=w401, "error in (no error)"=w400) -> ()  [unwired: 13 in, 1 out]
                  }
                  frame "Unknown", Default {
                    n196 = Search/Split String(string=w431, search string/char (-)=":") -> (substring before match=w429:string, match + rest of string=w427:string)  [unwired: 1 in, 1 out]
                    n197 = case shown="\"Video\"" w429 {
                      tunnel: [w432 w433 w451 w502 w532 w558 w568 w575 w582 w590 w660 w729 w799 w859 w882 w904] -> w422
                      tunnel: w428 -> [w432 w435 w443 w496 w525 w558 w568 w575 w582 w595 w664 w733 w803 w874 w895 w916]
                      tunnel: w427 -> [_ w436 w454 w505 w535 _ _ _ _ w596 w665 w734 w804 w875 w896 w917]
                      frame "Unknown", Default {
                      }
                      frame "Video" {
                        n198 = control-ref of="Capture"() -> (w434:refnum<vi>)
                        n199 = call "Video Select Source.vi"("Cluster In"=w435, "Source Name"=w436, "Bool Refnum"=w434) -> ("Cluster Out"=w433:T6)
                      }
                      frame "Audio" {
                        n200 = call "DirectShow - Enumerate Audio Devices.vi"() -> ("Devices"=w450:T3[], "Names"=w449:string[])  [unwired: 13 in, 1 out]
                        n201 = Search/Split String(string=w454, offset (0)=1) -> (match + rest of string=w452:string)  [unwired: 1 in, 2 out]
                        n202 = Search 1D Array(1D array=w449, element=w452) -> (index of element=w446:i32)  [unwired: 1 in]
                        n203 = Unbundle By Name(w443) -> ("IFilterGraph2"=w442:refnum<k24>, "Audio.Name"=w441:string)
                        n204 = Index Array(array=w450, index=w446) -> (element=w447:T3)
                        n205 = Less Than 0?(x=w446) -> (x < 0?=w445:bool)
                        n206 = Select(t=T3 {"DSDevice"=refnum, "DevicePath"="", "Mon"=refnum, "Name"=""}, s=w445, f=w447) -> (s? t:f=w438:T3)
                        n207 = case shown="False" w445 {
                          tunnel: w438 -> [w461 _]
                          tunnel: [w460 _] -> w444
                          tunnel: w442 -> [w459 w487]
                          tunnel: w441 -> [w457 w486]
                          tunnel: [w456 w484] -> w439
                          tunnel: [T4."Enabled" ("Disabled") T4."Disabled and Grayed Out" ("Disabled")] -> w437
                          frame False {
                            n208 = Empty String/Path?(string/path=w457) -> (empty?=w458:bool)
                            n209 = case shown="False" w458 {
                              tunnel: w461 -> [w467 w479]
                              tunnel: [w464 w476] -> w460
                              tunnel: w459 -> [w463 w473]
                              tunnel: w457 -> [_ w472]
                              tunnel: [w462 w471] -> w456
                              frame True {
                                n210 = call "DirectShow - Add Source Filter for Moniker.vi"("IFilterGraph2"=w463, "Device"=w467) -> ("IFilterGraph2 dup"=w462:refnum<k24>, "ppFilter"=w468:refnum<k24>, "error out"=w469:errorcluster)  [unwired: 11 in]
                                n211 = call "DirectShow - Find Pin ByCategory.vi"("Source"=w468, "Category"=T5."Capture", "error in (no error)"=w469) -> ("DS_Pin"=w465:refnum<k24>, "error out"=w466:errorcluster)  [unwired: 11 in]
                                n212 = call "DirectShow - Get Audio Stream Parameters.vi"("Stream"=w465, "error in (no error)"=w466) -> ("Abbreviated"=w464:string[])  [unwired: 9 in, 4 out]
                              }
                              frame False {
                                n213 = call "DirectShow - Delete Filter by Name.vi"("IFilterGraph2"=w473, "pName"=w472) -> ("IFilterGraph2 dup"=w475:refnum<k24>, "error out"=w474:errorcluster)  [unwired: 12 in]
                                n214 = call "DirectShow - Add Source Filter for Moniker.vi"("IFilterGraph2"=w475, "Device"=w479, "error in (no error)"=w474) -> ("IFilterGraph2 dup"=w471:refnum<k24>, "ppFilter"=w480:refnum<k24>, "error out"=w481:errorcluster)  [unwired: 10 in]
                                n215 = call "DirectShow - Find Pin ByCategory.vi"("Source"=w480, "Category"=T5."Capture", "error in (no error)"=w481) -> ("DS_Pin"=w477:refnum<k24>, "error out"=w478:errorcluster)  [unwired: 11 in]
                                n216 = call "DirectShow - Get Audio Stream Parameters.vi"("Stream"=w477, "error in (no error)"=w478) -> ("Abbreviated"=w476:string[])  [unwired: 9 in, 4 out]
                              }
                            }
                          }
                          frame True {
                            n217 = Empty String/Path?(string/path=w486) -> (empty?=w485:bool)
                            n218 = case shown="False" w485 {
                              tunnel: w487 -> [w490 w491]
                              tunnel: w486 -> [w489 _]
                              tunnel: [w488 w491] -> w484
                              frame False {
                                n219 = call "DirectShow - Delete Filter by Name.vi"("IFilterGraph2"=w490, "pName"=w489) -> ("IFilterGraph2 dup"=w488:refnum<k24>)  [unwired: 12 in, 1 out]
                              }
                              frame True {
                              }
                            }
                          }
                        }
                        n220 = call "DirectShow - Get Current Audio Format.vi"("IFilterGraph2"=w439, "Audio"=w438) -> ("Abbreviated"=w440:string)  [unwired: 10 in, 3 out]
                        n221 = property on="Capture" class="Bool (strict)"("DisabledEnum"=w437) -> ()  [unwired: 2 in, 2 out]
                        n222 = Bundle By Name(cluster=w443, "CurrentAudio"=w440, "Audio"=w438, "Audio Caps"=w444) -> (w451:T6)
                      }
                      frame "VideoC" {
                        n223 = call "DirectShow - Enumerate Video Compressors.vi"() -> ("Devices"=w501:T3[], "Names"=w500:string[])  [unwired: 13 in, 1 out]
                        n224 = Search/Split String(string=w505, offset (0)=1) -> (match + rest of string=w503:string)  [unwired: 1 in, 2 out]
                        n225 = Search 1D Array(1D array=w500, element=w503) -> (index of element=w498:i32)  [unwired: 1 in]
                        n226 = Unbundle By Name(w496) -> ("IFilterGraph2"=w495:refnum<k24>, "VideoC.Name"=w494:string)
                        n227 = Less Than 0?(x=w498) -> (x < 0?=w493:bool)
                        n228 = Index Array(array=w501, index=w498) -> (element=w497:T3)
                        n229 = Select(t=T3 {"DSDevice"=refnum, "DevicePath"="", "Mon"=refnum, "Name"=""}, s=w493, f=w497) -> (s? t:f=w492:T3)
                        n230 = case shown="False" w493 {
                          tunnel: w492 -> [w509 _]
                          tunnel: w495 -> [w508 w519]
                          tunnel: w494 -> [w506 w518]
                          frame False {
                            n231 = Empty String/Path?(string/path=w506) -> (empty?=w507:bool)
                            n232 = case shown="False" w507 {
                              tunnel: w509 -> [w511 w516]
                              tunnel: w508 -> [w510 w513]
                              tunnel: w506 -> [_ w512]
                              frame True {
                                n233 = call "DirectShow - Add Source Filter for Moniker.vi"("IFilterGraph2"=w510, "Device"=w511) -> ()  [unwired: 11 in, 3 out]
                              }
                              frame False {
                                n234 = call "DirectShow - Delete Filter by Name.vi"("IFilterGraph2"=w513, "pName"=w512) -> ("IFilterGraph2 dup"=w515:refnum<k24>, "error out"=w514:errorcluster)  [unwired: 12 in]
                                n235 = call "DirectShow - Add Source Filter for Moniker.vi"("IFilterGraph2"=w515, "Device"=w516, "error in (no error)"=w514) -> ()  [unwired: 10 in, 3 out]
                              }
                            }
                          }
                          frame True {
                            n236 = Empty String/Path?(string/path=w518) -> (empty?=w517:bool)
                            n237 = case shown="False" w517 {
                              tunnel: w519 -> [w521 _]
                              tunnel: w518 -> [w520 _]
                              frame False {
                                n238 = call "DirectShow - Delete Filter by Name.vi"("IFilterGraph2"=w521, "pName"=w520) -> ()  [unwired: 12 in, 2 out]
                              }
                              frame True {
                              }
                            }
                          }
                        }
                        n239 = Bundle By Name(cluster=w496, "VideoC"=w492) -> (w502:T6)
                      }
                      frame "AudioC" {
                        n240 = call "DirectShow - Enumerate Audio Compressors.vi"() -> ("Devices"=w531:T3[], "Names"=w530:string[])  [unwired: 13 in, 1 out]
                        n241 = Search/Split String(string=w535, offset (0)=1) -> (match + rest of string=w533:string)  [unwired: 1 in, 2 out]
                        n242 = Search 1D Array(1D array=w530, element=w533) -> (index of element=w528:i32)  [unwired: 1 in]
                        n243 = Unbundle By Name(w525) -> ("IFilterGraph2"=w523:refnum<k24>, "AudioC.Name"=w522:string)
                        n244 = Less Than 0?(x=w528) -> (x < 0?=w526:bool)
                        n245 = Index Array(array=w531, index=w528) -> (element=w527:T3)
                        n246 = Select(t=T3 {"DSDevice"=refnum, "DevicePath"="", "Mon"=refnum, "Name"=""}, s=w526, f=w527) -> (s? t:f=w524:T3)
                        n247 = case shown="False" w526 {
                          tunnel: w524 -> [w539 _]
                          tunnel: w523 -> [w538 w549]
                          tunnel: w522 -> [w536 w548]
                          frame False {
                            n248 = Empty String/Path?(string/path=w536) -> (empty?=w537:bool)
                            n249 = case shown="False" w537 {
                              tunnel: w539 -> [w541 w546]
                              tunnel: w538 -> [w540 w543]
                              tunnel: w536 -> [_ w542]
                              frame True {
                                n250 = call "DirectShow - Add Source Filter for Moniker.vi"("IFilterGraph2"=w540, "Device"=w541) -> ()  [unwired: 11 in, 3 out]
                              }
                              frame False {
                                n251 = call "DirectShow - Delete Filter by Name.vi"("IFilterGraph2"=w543, "pName"=w542) -> ("IFilterGraph2 dup"=w545:refnum<k24>, "error out"=w544:errorcluster)  [unwired: 12 in]
                                n252 = call "DirectShow - Add Source Filter for Moniker.vi"("IFilterGraph2"=w545, "Device"=w546, "error in (no error)"=w544) -> ()  [unwired: 10 in, 3 out]
                              }
                            }
                          }
                          frame True {
                            n253 = Empty String/Path?(string/path=w548) -> (empty?=w547:bool)
                            n254 = case shown="False" w547 {
                              tunnel: w549 -> [w551 _]
                              tunnel: w548 -> [w550 _]
                              frame False {
                                n255 = call "DirectShow - Delete Filter by Name.vi"("IFilterGraph2"=w551, "pName"=w550) -> ()  [unwired: 12 in, 2 out]
                              }
                              frame True {
                              }
                            }
                          }
                        }
                        n256 = Bundle By Name(cluster=w525, "AudioC"=w524) -> (w532:T6)
                      }
                      frame "Video Capture Device" {
                        n257 = Unbundle By Name(w558) -> ("IFilterGraph2"=w556:refnum<k24>, "Preview"=w557:refnum<k24>, "Video.Name"=w552:string, "Error"=w555:errorcluster)
                        n258 = call "DirectShow - Find Filter by Name.vi"("IFilterGraph2"=w556, "pName"=w552, "error in (no error)"=w555) -> ("ppFilter"=w553:refnum<k24>, "error out"=w554:errorcluster)  [unwired: 10 in, 1 out]
                        n259 = call "DirectShow - Property Dialog.vi"("IBaseFilter"=w553, "Owner"=w557, "Name"=w552, "error in (no error)"=w554) -> ()  [unwired: 11 in, 1 out]
                      }
                      frame "Video Capture Pin" {
                        n260 = Unbundle By Name(w568) -> ("IFilterGraph2"=w560:refnum<k24>, "Preview"=w567:refnum<k24>, "Video.Name"=w559:string, "Error"=w563:errorcluster)
                        n261 = call "DirectShow - Find Filter by Name.vi"("IFilterGraph2"=w560, "pName"=w559, "error in (no error)"=w563) -> ("ppFilter"=w561:refnum<k24>, "error out"=w562:errorcluster)  [unwired: 10 in, 1 out]
                        n262 = call "DirectShow - Find Pin ByCategory.vi"("Source"=w561, "Category"=T5."Capture", "error in (no error)"=w562) -> ("DS_Pin"=w564:refnum<k24>, "error out"=w565:errorcluster)  [unwired: 11 in]
                        n263 = call "DirectShow - Pin Property Page.vi"("DS_Pin"=w564, "Owner"=w567, "error in (no error)"=w565) -> ()  [unwired: 12 in, 1 out]
                      }
                      frame "Video Compressor" {
                        n264 = Unbundle By Name(w575) -> ("IFilterGraph2"=w571:refnum<k24>, "Preview"=w572:refnum<k24>, "VideoC.Name"=w569:string, "Error"=w570:errorcluster)
                        n265 = call "DirectShow - Find Filter by Name.vi"("IFilterGraph2"=w571, "pName"=w569, "error in (no error)"=w570) -> ("ppFilter"=w573:refnum<k24>, "error out"=w574:errorcluster)  [unwired: 10 in, 1 out]
                        n266 = call "DirectShow - Property Dialog.vi"("IBaseFilter"=w573, "Owner"=w572, "Name"=w569, "error in (no error)"=w574) -> ()  [unwired: 11 in, 1 out]
                      }
                      frame "Audio Capture Device" {
                        n267 = Unbundle By Name(w582) -> ("IFilterGraph2"=w579:refnum<k24>, "Preview"=w578:refnum<k24>, "Audio.Name"=w577:string, "Error"=w576:errorcluster)
                        n268 = call "DirectShow - Find Filter by Name.vi"("IFilterGraph2"=w579, "pName"=w577, "error in (no error)"=w576) -> ("ppFilter"=w580:refnum<k24>, "error out"=w581:errorcluster)  [unwired: 10 in, 1 out]
                        n269 = call "DirectShow - Property Dialog.vi"("IBaseFilter"=w580, "Owner"=w578, "Name"=w577, "error in (no error)"=w581) -> ()  [unwired: 11 in, 1 out]
                      }
                      frame "VideoFormat" {
                        n270 = Unbundle By Name(w595) -> ("Preview"=w585:refnum<k24>, "ScaleWindow?"=w587:bool, "Pane"=w586:refnum<vi>, "Preview?"=w588:bool, "FrameGrabber?"=w584:bool, "Audio"=w583:T3, "IFilterGraph2"=w592:refnum<k24>, "Video"=w591:T3, "CurrentVideo"=w593:string)
                        n271 = Search/Split String(string=w596, offset (0)=1) -> (match + rest of string=w594:string)  [unwired: 1 in, 2 out]
                        n272 = case shown="True" w588 {
                          tunnel: w594 -> [w609 w634]
                          tunnel: w593 -> [w607 w632]
                          tunnel: w592 -> [w603 w626]
                          tunnel: w591 -> [w599 w613]
                          tunnel: [w598 w619] -> w589
                          tunnel: w587 -> [_ w618]
                          tunnel: w586 -> [_ w617]
                          tunnel: w585 -> [_ w616]
                          tunnel: w584 -> [_ w614]
                          tunnel: w583 -> [_ w615]
                          frame False {
                            w606 = "%s %dx%d, %.2ffps, %dbit" ("format string")
                            n273 = Scan From String(format string=w606, input string=w607) -> (error out=w608:errorcluster, output 2=w612:i32, output 3=w611:i32, output 4=w610:dbl, output 5=w602:i32)  [unwired: 8 in, 2 out]
                            n274 = Format Into String(format string=w606, error in=w608, w609, w612, w611, w610, w602) -> (resulting string=w604:string, error out=w605:errorcluster)  [unwired: 1 in]
                            n275 = call "DirectShow - Set User Video Format.vi"("IFilterGraph2"=w603, "Video"=w599, "User Format"=w604, "error in (no error)"=w605) -> ("IFilterGraph2 dup"=w600:refnum<k24>, "error out"=w601:errorcluster)  [unwired: 10 in]
                            n276 = call "DirectShow - Get Current Video Format.vi"("IFilterGraph2"=w600, "Video"=w599, "error in (no error)"=w601) -> ("Abbreviated"=w598:string)  [unwired: 9 in, 3 out]
                          }
                          frame True {
                            w631 = "%s %dx%d, %.2ffps, %dbit" ("format string")
                            n277 = call "DirectShow - Media Control - Stop Preview.vi"("IFilterGraph2"=w626, "Video"=w613, "Audio"=w615, "FrameGrabber?"=w614) -> ("IFilterGraph2 dup"=w625:refnum<k24>, "error out"=w624:errorcluster)  [unwired: 10 in]
                            n278 = Scan From String(format string=w631, input string=w632) -> (error out=w633:errorcluster, output 2=w637:i32, output 3=w636:i32, output 4=w635:dbl, output 5=w629:i32)  [unwired: 8 in, 2 out]
                            n279 = Format Into String(format string=w631, error in=w633, w634, w637, w636, w635, w629) -> (resulting string=w630:string)  [unwired: 1 in, 1 out]
                            n280 = call "DirectShow - Set User Video Format.vi"("IFilterGraph2"=w625, "Video"=w613, "User Format"=w630, "error in (no error)"=w624) -> ("IFilterGraph2 dup"=w627:refnum<k24>, "error out"=w628:errorcluster)  [unwired: 10 in]
                            n281 = call "DirectShow - Get Current Video Format.vi"("IFilterGraph2"=w627, "Video"=w613, "error in (no error)"=w628) -> ("IFIlterGraph2 dup"=w623:refnum<k24>, "Abbreviated"=w619:string, "error out"=w622:errorcluster)  [unwired: 9 in, 1 out]
                            n282 = case shown="False" w618 {
                              tunnel: w617 -> [_ w644]
                              tunnel: [w638 w642] -> w621
                              tunnel: [w639 w643] -> w620
                              tunnel: w619 -> [w640 _]
                              frame False {
                                n283 = Scan From String(format string="%s %dx%d,%.2ffps,%dbit", input string=w640) -> (output 2=w638:i32, output 3=w639:i32)  [unwired: 10 in, 3 out]
                              }
                              frame True {
                                n284 = property class="Pane"(reference=w644) -> ("ContentBnds"=w649:T8)  [unwired: 1 in, 2 out]
                                n285 = Unbundle(w649) -> ("left"=w645:i16, "top"=w647:i16, "right"=w646:i16, "bottom"=w648:i16)
                                n286 = Subtract(x=w646, y=w645) -> (x-y=w642:i16)
                                n287 = Subtract(x=w648, y=w647) -> (x-y=w643:i16)
                              }
                            }
                            n288 = call "DirectShow - Media Control - Start Preview.vi"("IFilterGraph2"=w623, "PictureBox"=w616, "width"=w621, "height"=w620, "Video"=w613, "Audio"=w615, "FrameGrabber?"=w614, "error in (no error)"=w622) -> ()  [unwired: 6 in, 2 out]
                          }
                        }
                        n289 = Bundle By Name(cluster=w595, "CurrentVideo"=w589) -> (w590:T6)
                      }
                      frame "VideoRate" {
                        n290 = Unbundle By Name(w664) -> ("Preview"=w655:refnum<k24>, "ScaleWindow?"=w657:bool, "Pane"=w656:refnum<vi>, "Preview?"=w658:bool, "FrameGrabber?"=w654:bool, "Audio"=w653:T3, "IFilterGraph2"=w662:refnum<k24>, "Video"=w661:T3, "CurrentVideo"=w663:string)
                        n291 = Search/Split String(string=w665, offset (0)=1) -> (match + rest of string=w651:string)  [unwired: 1 in, 2 out]
                        n292 = Scan From String(format string="%.2f fps", input string=w651) -> (output 1=w650:dbl)  [unwired: 3 in, 3 out]
                        n293 = case shown="True" w658 {
                          tunnel: w663 -> [w678 w703]
                          tunnel: w662 -> [w674 w697]
                          tunnel: w661 -> [w670 w682]
                          tunnel: [w669 w690] -> w659
                          tunnel: w657 -> [_ w689]
                          tunnel: w656 -> [_ w688]
                          tunnel: w655 -> [_ w687]
                          tunnel: w654 -> [_ w685]
                          tunnel: w653 -> [_ w686]
                          tunnel: w650 -> [w667 w683]
                          frame False {
                            w677 = "%s %dx%d, %.2ffps, %dbit" ("format string")
                            n294 = Scan From String(format string=w677, input string=w678) -> (error out=w679:errorcluster, output 1=w668:string, output 2=w681:i32, output 3=w680:i32, output 5=w673:i32)  [unwired: 8 in, 2 out]
                            n295 = Format Into String(format string=w677, error in=w679, w668, w681, w680, w667, w673) -> (resulting string=w675:string, error out=w676:errorcluster)  [unwired: 1 in]
                            n296 = call "DirectShow - Set User Video Format.vi"("IFilterGraph2"=w674, "Video"=w670, "User Format"=w675, "error in (no error)"=w676) -> ("IFilterGraph2 dup"=w671:refnum<k24>, "error out"=w672:errorcluster)  [unwired: 10 in]
                            n297 = call "DirectShow - Get Current Video Format.vi"("IFilterGraph2"=w671, "Video"=w670, "error in (no error)"=w672) -> ("Abbreviated"=w669:string)  [unwired: 9 in, 3 out]
                          }
                          frame True {
                            w702 = "%s %dx%d, %.2ffps, %dbit" ("format string")
                            n298 = call "DirectShow - Media Control - Stop Preview.vi"("IFilterGraph2"=w697, "Video"=w682, "Audio"=w686, "FrameGrabber?"=w685) -> ("IFilterGraph2 dup"=w696:refnum<k24>, "error out"=w695:errorcluster)  [unwired: 10 in]
                            n299 = Scan From String(format string=w702, input string=w703) -> (error out=w704:errorcluster, output 1=w684:string, output 2=w706:i32, output 3=w705:i32, output 5=w700:i32)  [unwired: 8 in, 2 out]
                            n300 = Format Into String(format string=w702, error in=w704, w684, w706, w705, w683, w700) -> (resulting string=w701:string)  [unwired: 1 in, 1 out]
                            n301 = call "DirectShow - Set User Video Format.vi"("IFilterGraph2"=w696, "Video"=w682, "User Format"=w701, "error in (no error)"=w695) -> ("IFilterGraph2 dup"=w698:refnum<k24>, "error out"=w699:errorcluster)  [unwired: 10 in]
                            n302 = call "DirectShow - Get Current Video Format.vi"("IFilterGraph2"=w698, "Video"=w682, "error in (no error)"=w699) -> ("IFIlterGraph2 dup"=w694:refnum<k24>, "Abbreviated"=w690:string, "error out"=w693:errorcluster)  [unwired: 9 in, 1 out]
                            n303 = case shown="False" w689 {
                              tunnel: w688 -> [_ w713]
                              tunnel: [w707 w711] -> w692
                              tunnel: [w708 w712] -> w691
                              tunnel: w690 -> [w709 _]
                              frame False {
                                n304 = Scan From String(format string="%s %dx%d,%.2ffps,%dbit", input string=w709) -> (output 2=w707:i32, output 3=w708:i32)  [unwired: 10 in, 3 out]
                              }
                              frame True {
                                n305 = property class="Pane"(reference=w713) -> ("ContentBnds"=w718:T8)  [unwired: 1 in, 2 out]
                                n306 = Unbundle(w718) -> ("left"=w714:i16, "top"=w716:i16, "right"=w715:i16, "bottom"=w717:i16)
                                n307 = Subtract(x=w715, y=w714) -> (x-y=w711:i16)
                                n308 = Subtract(x=w717, y=w716) -> (x-y=w712:i16)
                              }
                            }
                            n309 = call "DirectShow - Media Control - Start Preview.vi"("IFilterGraph2"=w694, "PictureBox"=w687, "width"=w692, "height"=w691, "Video"=w682, "Audio"=w686, "FrameGrabber?"=w685, "error in (no error)"=w693) -> ()  [unwired: 6 in, 2 out]
                          }
                        }
                        n310 = Bundle By Name(cluster=w664, "CurrentVideo"=w659) -> (w660:T6)
                      }
                      frame "VideoBits" {
                        n311 = Unbundle By Name(w733) -> ("Preview"=w724:refnum<k24>, "ScaleWindow?"=w726:bool, "Pane"=w725:refnum<vi>, "Preview?"=w727:bool, "FrameGrabber?"=w723:bool, "Audio"=w722:T3, "IFilterGraph2"=w731:refnum<k24>, "Video"=w730:T3, "CurrentVideo"=w732:string)
                        n312 = Search/Split String(string=w734, offset (0)=1) -> (match + rest of string=w720:string)  [unwired: 1 in, 2 out]
                        n313 = Scan From String(format string="%d bit", input string=w720) -> (output 1=w719:i32)  [unwired: 3 in, 3 out]
                        n314 = case shown="True" w727 {
                          tunnel: w732 -> [w747 w772]
                          tunnel: w731 -> [w743 w767]
                          tunnel: w730 -> [w740 w753]
                          tunnel: [w739 w760] -> w728
                          tunnel: w726 -> [_ w759]
                          tunnel: w725 -> [_ w758]
                          tunnel: w724 -> [_ w757]
                          tunnel: w723 -> [_ w755]
                          tunnel: w722 -> [_ w756]
                          tunnel: w719 -> [w737 w752]
                          frame False {
                            w746 = "%s %dx%d, %.2ffps, %dbit" ("format string")
                            n315 = Scan From String(format string=w746, input string=w747) -> (error out=w748:errorcluster, output 1=w738:string, output 2=w750:i32, output 3=w749:i32, output 4=w736:dbl)  [unwired: 8 in, 2 out]
                            n316 = Format Into String(format string=w746, error in=w748, w738, w750, w749, w736, w737) -> (resulting string=w744:string, error out=w745:errorcluster)  [unwired: 1 in]
                            n317 = call "DirectShow - Set User Video Format.vi"("IFilterGraph2"=w743, "Video"=w740, "User Format"=w744, "error in (no error)"=w745) -> ("IFilterGraph2 dup"=w741:refnum<k24>, "error out"=w742:errorcluster)  [unwired: 10 in]
                            n318 = call "DirectShow - Get Current Video Format.vi"("IFilterGraph2"=w741, "Video"=w740, "error in (no error)"=w742) -> ("Abbreviated"=w739:string)  [unwired: 9 in, 3 out]
                          }
                          frame True {
                            w771 = "%s %dx%d, %.2ffps, %dbit" ("format string")
                            n319 = call "DirectShow - Media Control - Stop Preview.vi"("IFilterGraph2"=w767, "Video"=w753, "Audio"=w756, "FrameGrabber?"=w755) -> ("IFilterGraph2 dup"=w766:refnum<k24>, "error out"=w765:errorcluster)  [unwired: 10 in]
                            n320 = Scan From String(format string=w771, input string=w772) -> (error out=w773:errorcluster, output 1=w754:string, output 2=w775:i32, output 3=w774:i32, output 4=w751:dbl)  [unwired: 8 in, 2 out]
                            n321 = Format Into String(format string=w771, error in=w773, w754, w775, w774, w751, w752) -> (resulting string=w770:string)  [unwired: 1 in, 1 out]
                            n322 = call "DirectShow - Set User Video Format.vi"("IFilterGraph2"=w766, "Video"=w753, "User Format"=w770, "error in (no error)"=w765) -> ("IFilterGraph2 dup"=w768:refnum<k24>, "error out"=w769:errorcluster)  [unwired: 10 in]
                            n323 = call "DirectShow - Get Current Video Format.vi"("IFilterGraph2"=w768, "Video"=w753, "error in (no error)"=w769) -> ("IFIlterGraph2 dup"=w764:refnum<k24>, "Abbreviated"=w760:string, "error out"=w763:errorcluster)  [unwired: 9 in, 1 out]
                            n324 = case shown="False" w759 {
                              tunnel: w758 -> [_ w782]
                              tunnel: [w776 w780] -> w762
                              tunnel: [w777 w781] -> w761
                              tunnel: w760 -> [w778 _]
                              frame False {
                                n325 = Scan From String(format string="%s %dx%d,%.2ffps,%dbit", input string=w778) -> (output 2=w776:i32, output 3=w777:i32)  [unwired: 10 in, 3 out]
                              }
                              frame True {
                                n326 = property class="Pane"(reference=w782) -> ("ContentBnds"=w787:T8)  [unwired: 1 in, 2 out]
                                n327 = Unbundle(w787) -> ("left"=w783:i16, "top"=w785:i16, "right"=w784:i16, "bottom"=w786:i16)
                                n328 = Subtract(x=w784, y=w783) -> (x-y=w780:i16)
                                n329 = Subtract(x=w786, y=w785) -> (x-y=w781:i16)
                              }
                            }
                            n330 = call "DirectShow - Media Control - Start Preview.vi"("IFilterGraph2"=w764, "PictureBox"=w757, "width"=w762, "height"=w761, "Video"=w753, "Audio"=w756, "FrameGrabber?"=w755, "error in (no error)"=w763) -> ()  [unwired: 6 in, 2 out]
                          }
                        }
                        n331 = Bundle By Name(cluster=w733, "CurrentVideo"=w728) -> (w729:T6)
                      }
                      frame "VideoSize" {
                        n332 = Unbundle By Name(w803) -> ("Preview"=w794:refnum<k24>, "ScaleWindow?"=w796:bool, "Pane"=w795:refnum<vi>, "Preview?"=w797:bool, "FrameGrabber?"=w793:bool, "Audio"=w792:T3, "IFilterGraph2"=w801:refnum<k24>, "Video"=w800:T3, "CurrentVideo"=w802:string)
                        n333 = Search/Split String(string=w804, offset (0)=1) -> (match + rest of string=w791:string)  [unwired: 1 in, 2 out]
                        n334 = Scan From String(format string="%dx%d", input string=w791) -> (output 1=w790:i32, output 2=w788:i32)  [unwired: 4 in, 3 out]
                        n335 = case shown="True" w797 {
                          tunnel: w802 -> [w819 w844]
                          tunnel: w801 -> [w815 w839]
                          tunnel: w800 -> [w812 w825]
                          tunnel: [w811 w832] -> w798
                          tunnel: w796 -> [_ w831]
                          tunnel: w795 -> [_ w830]
                          tunnel: w794 -> [_ w829]
                          tunnel: w793 -> [_ w827]
                          tunnel: w792 -> [_ w828]
                          tunnel: w790 -> [w807 w821]
                          tunnel: w788 -> [w806 w822]
                          frame False {
                            w818 = "%s %dx%d, %.2ffps, %dbit" ("format string")
                            n336 = Scan From String(format string=w818, input string=w819) -> (error out=w820:errorcluster, output 1=w810:string, output 4=w809:dbl, output 5=w808:i32)  [unwired: 9 in, 2 out]
                            n337 = Format Into String(format string=w818, error in=w820, w810, w807, w806, w809, w808) -> (resulting string=w816:string, error out=w817:errorcluster)  [unwired: 1 in]
                            n338 = call "DirectShow - Set User Video Format.vi"("IFilterGraph2"=w815, "Video"=w812, "User Format"=w816, "error in (no error)"=w817) -> ("IFilterGraph2 dup"=w813:refnum<k24>, "error out"=w814:errorcluster)  [unwired: 10 in]
                            n339 = call "DirectShow - Get Current Video Format.vi"("IFilterGraph2"=w813, "Video"=w812, "error in (no error)"=w814) -> ("Abbreviated"=w811:string)  [unwired: 9 in, 3 out]
                          }
                          frame True {
                            w843 = "%s %dx%d, %.2ffps, %dbit" ("format string")
                            n340 = call "DirectShow - Media Control - Stop Preview.vi"("IFilterGraph2"=w839, "Video"=w825, "Audio"=w828, "FrameGrabber?"=w827) -> ("IFilterGraph2 dup"=w838:refnum<k24>, "error out"=w837:errorcluster)  [unwired: 10 in]
                            n341 = Scan From String(format string=w843, input string=w844) -> (error out=w845:errorcluster, output 1=w826:string, output 4=w824:dbl, output 5=w823:i32)  [unwired: 9 in, 2 out]
                            n342 = Format Into String(format string=w843, error in=w845, w826, w821, w822, w824, w823) -> (resulting string=w842:string)  [unwired: 1 in, 1 out]
                            n343 = call "DirectShow - Set User Video Format.vi"("IFilterGraph2"=w838, "Video"=w825, "User Format"=w842, "error in (no error)"=w837) -> ("IFilterGraph2 dup"=w840:refnum<k24>, "error out"=w841:errorcluster)  [unwired: 10 in]
                            n344 = call "DirectShow - Get Current Video Format.vi"("IFilterGraph2"=w840, "Video"=w825, "error in (no error)"=w841) -> ("IFIlterGraph2 dup"=w836:refnum<k24>, "Abbreviated"=w832:string, "error out"=w835:errorcluster)  [unwired: 9 in, 1 out]
                            n345 = case shown="False" w831 {
                              tunnel: w830 -> [_ w852]
                              tunnel: [w846 w850] -> w834
                              tunnel: [w847 w851] -> w833
                              tunnel: w832 -> [w848 _]
                              frame False {
                                n346 = Scan From String(format string="%s %dx%d,%.2ffps,%dbit", input string=w848) -> (output 2=w846:i32, output 3=w847:i32)  [unwired: 10 in, 3 out]
                              }
                              frame True {
                                n347 = property class="Pane"(reference=w852) -> ("ContentBnds"=w857:T8)  [unwired: 1 in, 2 out]
                                n348 = Unbundle(w857) -> ("left"=w853:i16, "top"=w855:i16, "right"=w854:i16, "bottom"=w856:i16)
                                n349 = Subtract(x=w854, y=w853) -> (x-y=w850:i16)
                                n350 = Subtract(x=w856, y=w855) -> (x-y=w851:i16)
                              }
                            }
                            n351 = call "DirectShow - Media Control - Start Preview.vi"("IFilterGraph2"=w836, "PictureBox"=w829, "width"=w834, "height"=w833, "Video"=w825, "Audio"=w828, "FrameGrabber?"=w827, "error in (no error)"=w835) -> ()  [unwired: 6 in, 2 out]
                          }
                        }
                        n352 = Bundle By Name(cluster=w803, "CurrentVideo"=w798) -> (w799:T6)
                      }
                      frame "AudioChan" {
                        n353 = Unbundle By Name(w874) -> ("IFilterGraph2"=w864:refnum<k24>, "Audio"=w860:T3, "CurrentAudio"=w869:string)
                        n354 = Search/Split String(string=w875, offset (0)=1) -> (match + rest of string=w865:string)  [unwired: 1 in, 2 out]
                        n355 = Search/Split String(string=w869, search string/char (-)=",") -> (match + rest of string=w872:string)  [unwired: 1 in, 2 out]
                        n356 = Scan From String(format string="%f kHz, %d bits", input string=w872, initial scan location=u32 2) -> (output 1=w867:dbl, output 2=w866:i32)  [unwired: 3 in, 3 out]
                        n357 = Format Into String(format string="%s, %.3f kHz, %d bits", w865, w867, w866) -> (resulting string=w863:string)  [unwired: 2 in, 1 out]
                        n358 = call "DirectShow - Set User Audio Format.vi"("IFilterGraph2"=w864, "Audio"=w860, "User Format"=w863) -> ("IFilterGraph2 dup"=w862:refnum<k24>, "error out"=w861:errorcluster)  [unwired: 11 in]
                        n359 = call "DirectShow - Get Current Audio Format.vi"("IFilterGraph2"=w862, "Audio"=w860, "error in (no error)"=w861) -> ("Abbreviated"=w858:string)  [unwired: 9 in, 3 out]
                        n360 = Bundle By Name(cluster=w874, "CurrentAudio"=w858) -> (w859:T6)
                      }
                      frame "AudioRate" {
                        n361 = Unbundle By Name(w895) -> ("IFilterGraph2"=w887:refnum<k24>, "Audio"=w883:T3, "CurrentAudio"=w890:string)
                        n362 = Search/Split String(string=w896, offset (0)=1) -> (match + rest of string=w879:string)  [unwired: 1 in, 2 out]
                        n363 = Scan From String(format string="%f kHz", input string=w879) -> (output 1=w877:dbl)  [unwired: 3 in, 3 out]
                        n364 = Search/Split String(string=w890, search string/char (-)=",") -> (substring before match=w878:string, match + rest of string=w893:string)  [unwired: 1 in, 1 out]
                        n365 = Scan From String(format string="%f kHz, %d bits", input string=w893, initial scan location=u32 2) -> (output 2=w888:i32)  [unwired: 4 in, 3 out]
                        n366 = Format Into String(format string="%s, %.3f kHz, %d bits", w878, w877, w888) -> (resulting string=w886:string)  [unwired: 2 in, 1 out]
                        n367 = call "DirectShow - Set User Audio Format.vi"("IFilterGraph2"=w887, "Audio"=w883, "User Format"=w886) -> ("IFilterGraph2 dup"=w885:refnum<k24>, "error out"=w884:errorcluster)  [unwired: 11 in]
                        n368 = call "DirectShow - Get Current Audio Format.vi"("IFilterGraph2"=w885, "Audio"=w883, "error in (no error)"=w884) -> ("Abbreviated"=w881:string)  [unwired: 9 in, 3 out]
                        n369 = Bundle By Name(cluster=w895, "CurrentAudio"=w881) -> (w882:T6)
                      }
                      frame "AudioSize" {
                        n370 = Unbundle By Name(w916) -> ("IFilterGraph2"=w909:refnum<k24>, "Audio"=w905:T3, "CurrentAudio"=w911:string)
                        n371 = Search/Split String(string=w917, offset (0)=1) -> (match + rest of string=w901:string)  [unwired: 1 in, 2 out]
                        n372 = Scan From String(format string="%d bits", input string=w901) -> (output 1=w899:i32)  [unwired: 3 in, 3 out]
                        n373 = Search/Split String(string=w911, search string/char (-)=",") -> (substring before match=w900:string, match + rest of string=w914:string)  [unwired: 1 in, 1 out]
                        n374 = Scan From String(format string="%f kHz, %d bits", input string=w914, initial scan location=u32 2) -> (output 1=w898:dbl)  [unwired: 4 in, 3 out]
                        n375 = Format Into String(format string="%s, %.3f kHz, %d bits", w900, w898, w899) -> (resulting string=w908:string)  [unwired: 2 in, 1 out]
                        n376 = call "DirectShow - Set User Audio Format.vi"("IFilterGraph2"=w909, "Audio"=w905, "User Format"=w908) -> ("IFilterGraph2 dup"=w907:refnum<k24>, "error out"=w906:errorcluster)  [unwired: 11 in]
                        n377 = call "DirectShow - Get Current Audio Format.vi"("IFilterGraph2"=w907, "Audio"=w905, "error in (no error)"=w906) -> ("Abbreviated"=w903:string)  [unwired: 9 in, 3 out]
                        n378 = Bundle By Name(cluster=w916, "CurrentAudio"=w903) -> (w904:T6)
                      }
                    }
                    n379 = Unbundle By Name(w422) -> ("Video Caps"=w424:string[], "CurrentVideo"=w423:string)
                    n380 = property on="Selector" class="Ring (strict)"("Strings []"=w424) -> (error out=w425:errorcluster)  [unwired: 2 in, 1 out]
                    n381 = Search 1D Array(1D array=w424, element=w423) -> (index of element=w426:i32)  [unwired: 1 in]
                    n382 = property on="Selector" class="Ring (strict)"(error in=w425, "Value"=w426) -> ()  [unwired: 1 in, 2 out]
                  }
                  frame "Preview" {
                    n383 = Get Menu Item Info(7:w928, 11:w931) -> (3:w929:refnum<k9>, 4:w922:bool)  [unwired: 1 in, 5 out]
                    n384 = Not(x=w922) -> (.not. x?=w921:bool)
                    n385 = Set Menu Item Info(6:w921, 7:w928, 9:TRUE ("enabled"), 11:w929) -> ()  [unwired: 3 in, 2 out]
                    n386 = control-ref of="Info"() -> (w927:refnum<vi>)
                    n387 = control-ref of="Stop"() -> (w926:refnum<vi>)
                    n388 = control-ref of="Run"() -> (w925:refnum<vi>)
                    n389 = control-ref of="Pause"() -> (w924:refnum<vi>)
                    n390 = control-ref of="Grab Window Image"() -> (w923:refnum<vi>)
                    n391 = call "Start Preview.vi"("Cluster In"=w920, "Start?"=w921, "Info"=w927, "Stop"=w926, "Pause"=w924, "Run"=w925, "Grab Window Image"=w923) -> ("Cluster Out"=w919:T6)  [unwired: 1 in]
                  }
                  frame "Enable Frame Grabber" {
                    n392 = Get Menu Item Info(7:w935, 11:w940) -> (3:w934:refnum<k9>, 4:w938:bool)  [unwired: 1 in, 5 out]
                    n393 = Not(x=w938) -> (.not. x?=w933:bool)
                    n394 = Set Menu Item Info(6:w933, 7:w935, 9:TRUE ("enabled"), 11:w934) -> ()  [unwired: 3 in, 2 out]
                    n395 = control-ref of="Grab Frame"() -> (w939:refnum<vi>)
                    n396 = call "Start Framegrabber.vi"("Cluster In"=w932, "Enable?"=w933, "Bool Refnum"=w939) -> ("Cluster Out"=w936:T6)
                  }
                  frame "Video Capabilities" {
                    n397 = Unbundle By Name(w945) -> ("Video.DevicePath"=w944:string, "Audio.DevicePath"=w943:string)
                    n398 = call "DirectShow - Get Capture Capabilities.vi"("VideoMoniker(DevicePath)"=w944, "AudioMoniker(DevicePath)"=w943) -> ("Video Device Capabilities"=w942:string, "error out"=w941:errorcluster)  [unwired: 11 in, 1 out]
                    n399 = call <vilib>:"Clear Errors.vi"("error in (no error)"=w941) -> ()  [unwired: 6 in, 1 out]
                    n400 = One Button Dialog(message=w942) -> ()  [unwired: 1 in, 1 out]
                  }
                  frame "Audio Capabilities" {
                    n401 = Unbundle By Name(w950) -> ("Video.DevicePath"=w949:string, "Audio.DevicePath"=w948:string)
                    n402 = call "DirectShow - Get Capture Capabilities.vi"("VideoMoniker(DevicePath)"=w949, "AudioMoniker(DevicePath)"=w948) -> ("Audio Device Capabilities"=w946:string, "error out"=w947:errorcluster)  [unwired: 11 in, 1 out]
                    n403 = call <vilib>:"Clear Errors.vi"("error in (no error)"=w947) -> ()  [unwired: 6 in, 1 out]
                    n404 = One Button Dialog(message=w946) -> ()  [unwired: 1 in, 1 out]
                  }
                  frame "Video Renderer Stats" {
                    w952 = "Renderer" ("Name")
                    n405 = Unbundle By Name(w972) -> ("IFilterGraph2"=w971:refnum<k24>)
                    n406 = call "DirectShow - Find Filter by Name.vi"("IFilterGraph2"=w971, "pName"=w952) -> ("ppFilter"=w951:refnum<k24>, "error out"=w965:errorcluster)  [unwired: 11 in, 1 out]
                    n407 = vi-ref "DirectShow - Property Dialog.vi"() -> (w967:refnum<vi>)
                    n408 = property class="VI"(reference=w967, error in=w965) -> (error out=w969:errorcluster, "Name"=w968:string)  [unwired: 1 out]
                    n409 = vi-ref "DirectShow - Property Dialog.vi"() -> (w966:refnum<vi>)
                    n410 = Open VI Reference(type specifier VI Refnum (for type only)=w966, vi path=w968, options=128, error in (no error)=w969) -> (vi reference=w953:refnum<vi>)  [unwired: 2 in, 1 out]
                    n411 = invoke class="VI Interface Type 0" method="Ctrl Val.Set"(reference=w953, "Control Name"="IBaseFilter", "Value"=w951) -> (reference out=w957:refnum<vi>, error out=w956:errorcluster)  [unwired: 2 in, 3 out]
                    n412 = invoke class="VI Interface Type 0" method="Ctrl Val.Set"(reference=w957, error in=w956, "Control Name"="Name", "Value"=w952) -> (reference out=w959:refnum<vi>, error out=w958:errorcluster)  [unwired: 1 in, 3 out]
                    n413 = invoke on="Invoke Node" class="VI Interface Type 0" method="FP.Open"(reference=w959, error in=w958, "Activate"=TRUE ("Activate?")) -> (reference out=w961:refnum<vi>, error out=w960:errorcluster)  [unwired: 2 in, 3 out]
                    n414 = invoke on="Invoke Node" class="VI Interface Type 0" method="Run VI"(reference=w961, error in=w960, "Wait until done"=FALSE ("Wait Until Done"), "Auto Dispose Ref"=TRUE ("Auto Dispose Reference")) -> ()  [unwired: 1 in, 5 out]
                  }
                  frame "Audio Renderer Stats" {
                    w973 = "AudioRenderer" ("Name")
                    n415 = Unbundle By Name(w994) -> ("IFilterGraph2"=w987:refnum<k24>)
                    n416 = call "DirectShow - Find Filter by Name.vi"("IFilterGraph2"=w987, "pName"=w973) -> ("ppFilter"=w974:refnum<k24>, "error out"=w988:errorcluster)  [unwired: 11 in, 1 out]
                    n417 = vi-ref "DirectShow - Property Dialog.vi"() -> (w990:refnum<vi>)
                    n418 = property class="VI"(reference=w990, error in=w988) -> (error out=w992:errorcluster, "Name"=w991:string)  [unwired: 1 out]
                    n419 = vi-ref "DirectShow - Property Dialog.vi"() -> (w989:refnum<vi>)
                    n420 = Open VI Reference(type specifier VI Refnum (for type only)=w989, vi path=w991, options=128, error in (no error)=w992) -> (vi reference=w977:refnum<vi>)  [unwired: 2 in, 1 out]
                    n421 = invoke class="VI Interface Type 0" method="Ctrl Val.Set"(reference=w977, "Control Name"="IBaseFilter", "Value"=w974) -> (reference out=w979:refnum<vi>, error out=w978:errorcluster)  [unwired: 2 in, 3 out]
                    n422 = invoke class="VI Interface Type 0" method="Ctrl Val.Set"(reference=w979, error in=w978, "Control Name"="Name", "Value"=w973) -> (reference out=w981:refnum<vi>, error out=w980:errorcluster)  [unwired: 1 in, 3 out]
                    n423 = invoke on="Invoke Node" class="VI Interface Type 0" method="FP.Open"(reference=w981, error in=w980, "Activate"=TRUE ("Activate?")) -> (reference out=w983:refnum<vi>, error out=w982:errorcluster)  [unwired: 2 in, 3 out]
                    n424 = invoke on="Invoke Node" class="VI Interface Type 0" method="Run VI"(reference=w983, error in=w982, "Wait until done"=FALSE ("Wait Until Done"), "Auto Dispose Ref"=TRUE ("Auto Dispose Reference")) -> ()  [unwired: 1 in, 5 out]
                  }
                }
              }
              event "Selector": Value Change {
                n425 = event-data() -> ("NewVal"=w998:u16)  [unwired: 1 in, 1 out]
                n426 = Greater Or Equal To 0?(x=w998) -> (x >= 0?=w997:bool)
                n427 = case shown="True" w997 {
                  tunnel: w998 -> [_ w1003]
                  tunnel: ["" w1002] -> w995
                  frame False {
                  }
                  frame True {
                    n428 = property on="Selector" class="Ring (strict)"() -> ("Strings []"=w1004:string[])  [unwired: 2 in, 2 out]
                    n429 = Index Array(array=w1004, index=w1003) -> (element=w1002:string)
                  }
                }
                n430 = Empty String/Path?(string/path=w995) -> (empty?=w996:bool)
                n431 = case shown="False" w996 {
                  tunnel: w1000 -> [w1010 w1071]
                  tunnel: [w1009 w1071] -> w999
                  tunnel: w995 -> [w1008 _]
                  frame False {
                    n432 = Unbundle By Name(w1010) -> ("Preview"=w1013:refnum<k24>, "ScaleWindow?"=w1015:bool, "Pane"=w1014:refnum<vi>, "Preview?"=w1016:bool, "FrameGrabber?"=w1012:bool, "Audio"=w1011:T3, "IFilterGraph2"=w1018:refnum<k24>, "Video"=w1017:T3)
                    n433 = case shown="True" w1016 {
                      tunnel: w1008 -> [w1030 w1055]
                      tunnel: w1018 -> [w1026 w1050]
                      tunnel: w1017 -> [w1023 w1036]
                      tunnel: [w1022 w1043] -> w1007
                      tunnel: w1015 -> [_ w1042]
                      tunnel: w1014 -> [_ w1041]
                      tunnel: w1013 -> [_ w1040]
                      tunnel: w1012 -> [_ w1038]
                      tunnel: w1011 -> [_ w1039]
                      frame False {
                        w1029 = "%s %dx%d, %.2ffps, %dbit" ("format string")
                        n434 = Scan From String(format string=w1029, input string=w1030) -> (error out=w1031:errorcluster, output 1=w1021:string, output 2=w1033:i32, output 3=w1032:i32, output 4=w1020:dbl, output 5=w1019:i32)  [unwired: 7 in, 2 out]
                        n435 = Format Into String(format string=w1029, error in=w1031, w1021, w1033, w1032, w1020, w1019) -> (resulting string=w1027:string, error out=w1028:errorcluster)  [unwired: 1 in]
                        n436 = call "DirectShow - Set User Video Format.vi"("IFilterGraph2"=w1026, "Video"=w1023, "User Format"=w1027, "error in (no error)"=w1028) -> ("IFilterGraph2 dup"=w1024:refnum<k24>, "error out"=w1025:errorcluster)  [unwired: 10 in]
                        n437 = call "DirectShow - Get Current Video Format.vi"("IFilterGraph2"=w1024, "Video"=w1023, "error in (no error)"=w1025) -> ("Abbreviated"=w1022:string)  [unwired: 9 in, 3 out]
                      }
                      frame True {
                        w1054 = "%s %dx%d, %.2ffps, %dbit" ("format string")
                        n438 = call "DirectShow - Media Control - Stop Preview.vi"("IFilterGraph2"=w1050, "Video"=w1036, "Audio"=w1039, "FrameGrabber?"=w1038) -> ("IFilterGraph2 dup"=w1049:refnum<k24>, "error out"=w1048:errorcluster)  [unwired: 10 in]
                        n439 = Scan From String(format string=w1054, input string=w1055) -> (error out=w1056:errorcluster, output 1=w1037:string, output 2=w1058:i32, output 3=w1057:i32, output 4=w1035:dbl, output 5=w1034:i32)  [unwired: 7 in, 2 out]
                        n440 = Format Into String(format string=w1054, error in=w1056, w1037, w1058, w1057, w1035, w1034) -> (resulting string=w1053:string)  [unwired: 1 in, 1 out]
                        n441 = call "DirectShow - Set User Video Format.vi"("IFilterGraph2"=w1049, "Video"=w1036, "User Format"=w1053, "error in (no error)"=w1048) -> ("IFilterGraph2 dup"=w1051:refnum<k24>, "error out"=w1052:errorcluster)  [unwired: 10 in]
                        n442 = call "DirectShow - Get Current Video Format.vi"("IFilterGraph2"=w1051, "Video"=w1036, "error in (no error)"=w1052) -> ("IFIlterGraph2 dup"=w1047:refnum<k24>, "Abbreviated"=w1043:string, "error out"=w1046:errorcluster)  [unwired: 9 in, 1 out]
                        n443 = case shown="False" w1042 {
                          tunnel: w1041 -> [_ w1065]
                          tunnel: [w1059 w1063] -> w1045
                          tunnel: [w1060 w1064] -> w1044
                          tunnel: w1043 -> [w1061 _]
                          frame False {
                            n444 = Scan From String(format string="%s %dx%d,%.2ffps,%dbit", input string=w1061) -> (output 2=w1059:i32, output 3=w1060:i32)  [unwired: 10 in, 3 out]
                          }
                          frame True {
                            n445 = property class="Pane"(reference=w1065) -> ("ContentBnds"=w1070:T8)  [unwired: 1 in, 2 out]
                            n446 = Unbundle(w1070) -> ("left"=w1066:i16, "top"=w1068:i16, "right"=w1067:i16, "bottom"=w1069:i16)
                            n447 = Subtract(x=w1067, y=w1066) -> (x-y=w1063:i16)
                            n448 = Subtract(x=w1069, y=w1068) -> (x-y=w1064:i16)
                          }
                        }
                        n449 = call "DirectShow - Media Control - Start Preview.vi"("IFilterGraph2"=w1047, "PictureBox"=w1040, "width"=w1045, "height"=w1044, "Video"=w1036, "Audio"=w1039, "FrameGrabber?"=w1038, "error in (no error)"=w1046) -> ()  [unwired: 6 in, 2 out]
                      }
                    }
                    n450 = Empty String/Path?(string/path=w1007) -> (empty?=w1006:bool)
                    n451 = Bundle By Name(cluster=w1010, "CurrentVideo"=w1007) -> (w1009:T6)
                    n452 = Not(x=w1006) -> (.not. x?=w1005:bool)
                    n453 = property on="Fit Window" class="Bool (strict)"("Val(Sgnl)"=w1005) -> ()  [unwired: 2 in, 2 out]
                  }
                  frame True {
                  }
                }
              }
              event "Fit Window": Value Change {
                n454 = event-data() -> ("NewVal"=w1072:bool)  [unwired: 1 in]
                n455 = Unbundle By Name(w1077) -> ("IFilterGraph2"=w1075:refnum<k24>, "Preview?"=w1076:bool, "Pane"=w1074:refnum<vi>, "CurrentVideo"=w1073:string)
                n456 = case shown="True" w1076 {
                  tunnel: w1075 -> [_ w1086]
                  tunnel: w1074 -> [_ w1088]
                  tunnel: w1073 -> [_ w1087]
                  tunnel: w1072 -> [_ w1079]
                  frame False {
                  }
                  frame True {
                    w1082 = 0 ("left")
                    w1085 = refnum<k24> refnum  # IVideoWindow
                    n457 = case shown="True" w1079 {
                      tunnel: w1088 -> [_ w1095]
                      tunnel: [w1090 w1094] -> w1080
                      tunnel: [w1091 w1093] -> w1081
                      tunnel: w1087 -> [w1089 _]
                      frame False {
                        n458 = Scan From String(format string="%s %dx%d,%.2ffps,%dbit", input string=w1089) -> (output 2=w1091:i32, output 3=w1090:i32)  [unwired: 10 in, 3 out]
                      }
                      frame True {
                        n459 = property class="Pane"(reference=w1095) -> ("ContentBnds"=w1100:T8)  [unwired: 1 in, 2 out]
                        n460 = Unbundle(w1100) -> ("left"=w1096:i16, "top"=w1098:i16, "right"=w1097:i16, "bottom"=w1099:i16)
                        n461 = Subtract(x=w1097, y=w1096) -> (x-y=w1093:i16)
                        n462 = Subtract(x=w1099, y=w1098) -> (x-y=w1094:i16)
                      }
                    }
                    n463 = To More Specific Class(target class=w1085, reference=w1086) -> (specific class reference=w1084:refnum<k24>, error out=w1083:errorcluster)  [unwired: 1 in]
                    n464 = invoke class="IVideoWindow" method="SetWindowPosition"(reference=w1084, error in=w1083, "left"=w1082, "top"=w1082, "width"=w1081, "height"=w1080) -> ()  [unwired: 1 in, 7 out]
                  }
                }
                n465 = Bundle By Name(cluster=w1077, "ScaleWindow?"=w1072) -> (w1078:T6)
              }
              event "Stop", "Run", "Pause": Value Change {
                n466 = event-data() -> ("CtlRef"=w1106:refnum<vi>)  [unwired: 1 in]
                n467 = property class="Bool"(reference=w1106) -> (reference out=w1104:refnum<vi>, error out=w1105:errorcluster, "Label.Text"=w1103:string)  [unwired: 1 in]
                n468 = Close Reference(reference=w1104, error in (no error)=w1105) -> ()  [unwired: 1 out]
                n469 = case shown="\"Pause\"" w1103 {
                  tunnel: [w1108 w1113 w1118 w1123] -> w1102
                  tunnel: w1101 -> [w1109 w1114 w1119 w1124]
                  frame "Unknown", Default {
                    n470 = Bundle By Name(cluster=w1109, "MediaState"=DirectShow_-_Media_State."Stopped") -> (w1108:T6)
                  }
                  frame "Stop" {
                    n471 = Unbundle By Name(w1114) -> ("IFilterGraph2"=w1111:refnum<k24>)  [unwired: 1 out]
                    n472 = call "DirectShow - Media Control - StartStopPause.vi"("IFilterGraph2"=w1111, "Mode"=DirectShow_-_Media_Mode."Stop") -> ()  [unwired: 12 in, 2 out]
                    n473 = Bundle By Name(cluster=w1114, "MediaState"=DirectShow_-_Media_State."Stopped") -> (w1113:T6)
                  }
                  frame "Run" {
                    n474 = Unbundle By Name(w1119) -> ("IFilterGraph2"=w1116:refnum<k24>)  [unwired: 1 out]
                    n475 = call "DirectShow - Media Control - StartStopPause.vi"("IFilterGraph2"=w1116, "Mode"=DirectShow_-_Media_Mode."Run") -> ()  [unwired: 12 in, 2 out]
                    n476 = Bundle By Name(cluster=w1119, "MediaState"=DirectShow_-_Media_State."Playing") -> (w1118:T6)
                  }
                  frame "Pause" {
                    n477 = Unbundle By Name(w1124) -> ("IFilterGraph2"=w1121:refnum<k24>)  [unwired: 1 out]
                    n478 = call "DirectShow - Media Control - StartStopPause.vi"("IFilterGraph2"=w1121, "Mode"=DirectShow_-_Media_Mode."Pause") -> ()  [unwired: 12 in, 2 out]
                    n479 = Bundle By Name(cluster=w1124, "MediaState"=DirectShow_-_Media_State."Paused") -> (w1123:T6)
                  }
                }
              }
              event "Grab Frame": Value Change {
                w1125 = FALSE ("Snapshot")
                n480 = event-data() -> ()  [unwired: 1 in, 1 out]
                n481 = Unbundle By Name(w1126) -> ("FrameGrab"=w1131:refnum<k24>, "IFilterGraph2"=w1130:refnum<k24>, "CurrentVideo"=w1132:string, "FrameGrabber?"=w1129:bool, "Preview?"=w1128:bool)
                n482 = And(x=w1129, y=w1128) -> (x .and. y?=w1127:bool)
                n483 = case shown="True" w1127 {
                  tunnel: w1132 -> [_ w1152]
                  tunnel: w1131 -> [_ w1133]
                  tunnel: w1130 -> [_ w1151]
                  frame False {
                  }
                  frame True {
                    w1150 = refnum<k24> refnum  # ISampleGrabber
                    n484 = Scan From String(format string="%s %dx%d,%.2ffps,%dbit", input string=w1152) -> (output 2=w1140:i32, output 3=w1141:i32)  [unwired: 10 in, 3 out]
                    n485 = call "DirectShow - Find Filter by Name.vi"("IFilterGraph2"=w1151, "pName"="Grabber") -> ("ppFilter"=w1144:refnum<k24>, "error out"=w1145:errorcluster)  [unwired: 11 in, 1 out]
                    n486 = To More Specific Class(target class=w1150, reference=w1144, error in=w1145) -> (specific class reference=w1139:refnum<k24>, error out=w1142:errorcluster)
                    n487 = local read "Capture Folder"() -> (w1138:path)
                    n488 = call "DirectShow - SampleGrabber Snap (JPEG).vi"("ISampleGrabber"=w1139, "width"=w1140, "height"=w1141, "error in"=w1142) -> ("Bitmap"=w1134:refnum<k24>)  [unwired: 9 in, 2 out]
                    n489 = call "Build File Name.vi"("Folder"=w1138, "Extension"="jpg") -> ("Path Out"=w1135:path, "File Path String"=w1136:string, "Error"=w1137:errorcluster)  [unwired: 2 in, 1 out]
                    n490 = case shown="No Error" w1137 {
                      tunnel: w1136 -> [w1159 _]
                      tunnel: w1134 -> [w1158 _]
                      tunnel: w1135 -> [w1157 _]
                      tunnel: w1133 -> [w1156 _]
                      frame No Error {
                        w1155 = 1 items=["Normal", "StretchImage", "AutoSize", "CenterImage", "Zoom"] ("SizeMode")
                        n491 = local write "Capture Folder"(w1157) -> ()
                        n492 = invoke class="Bitmap" method="Save"(reference=w1158, "filename"=w1159) -> (reference out=w1154:refnum<k24>)  [unwired: 2 in, 3 out]
                        n493 = property class="PictureBox"(reference=w1156, "Image"=w1154, "SizeMode"=w1155) -> ()  [unwired: 1 in, 2 out]
                      }
                      frame Error {
                        n494 = call "Display Message to User2"() -> ()  [unwired: 10 in, 2 out]
                      }
                    }
                    n495 = Get Date/Time In Seconds() -> (seconds since 1Jan1904=w1147:timestamp)
                    n496 = Format Into String(format string="%<%H:%M:%S%.3u %p>T\nFormat:     24-bit RGB\nSize:               %d x%d", w1147, w1140, w1141) -> (resulting string=→"Summary":string)  [unwired: 2 in, 1 out]
                  }
                }
                n497 = local write "Grab Frame"(w1125) -> ()
                n498 = global write "Remote Snapshot.vi" "Snapshot"(w1125) -> ()
              }
              event "Grab Window Image": Value Change {
                n499 = event-data() -> ()  [unwired: 1 in, 1 out]
                n500 = Unbundle By Name(w1160) -> ("WindowSnap"=w1162:refnum<k24>, "IFilterGraph2"=w1163:refnum<k24>, "Preview?"=w1161:bool)
                n501 = case shown="True" w1161 {
                  tunnel: w1163 -> [_ w1181]
                  tunnel: w1162 -> [_ w1171]
                  frame False {
                  }
                  frame True {
                    w1178 = refnum<k24> refnum  # IBasicVideo2
                    w1180 = refnum<k24> refnum  # IMediaControl
                    n502 = To More Specific Class(target class=w1180, reference=w1181) -> (specific class reference=w1179:refnum<k24>, error out=w1177:errorcluster)  [unwired: 1 in]
                    n503 = invoke class="IMediaControl" method="Pause"(reference=w1179, error in=w1177) -> (reference out=w1170:refnum<k24>, error out=w1176:errorcluster)  [unwired: 1 in, 1 out]
                    n504 = To More Specific Class(target class=w1178, reference=w1170, error in=w1176) -> (specific class reference=w1174:refnum<k24>, error out=w1175:errorcluster)
                    n505 = invoke class="IBasicVideo2" method="GetVideoSize"(reference=w1174, error in=w1175) -> (reference out=w1173:refnum<k24>, error out=w1172:errorcluster, "pWidth"=w1167:i32, "pHeight"=w1166:i32)  [unwired: 3 in, 1 out]
                    n506 = Get Date/Time In Seconds() -> (seconds since 1Jan1904=w1168:timestamp)
                    n507 = Format Into String(format string="%<%I:%M:%S%.3u %p>T\nFormat:    32-bit RGB\nSize:               %d x%d", w1168, w1167, w1166) -> (resulting string=→"SnapSummary":string)  [unwired: 2 in, 1 out]
                    n508 = call "DirectShow - Picture Snap (DIB Image).vi"("IBasicVideo2"=w1173, "Snap"=w1171, "error in (no error)"=w1172) -> ("error out"=w1164:errorcluster)  [unwired: 11 in, 1 out]
                    n509 = invoke class="IMediaControl" method="Run"(reference=w1170, error in=w1164) -> ()  [unwired: 1 in, 3 out]
                  }
                }
              }
              event "Capture": Value Change {
                n510 = event-data() -> ("NewVal"=w1184:bool)  [unwired: 1 in]
                n511 = case shown="True" w1184 {
                  tunnel: [w1204 w1241] -> w1183
                  tunnel: w1182 -> [w1202 w1240]
                  frame False {
                    n512 = Unbundle By Name(w1202) -> ("Preview"=w1197:refnum<k24>, "ScaleWindow?"=w1200:bool, "Pane"=w1199:refnum<vi>, "CurrentVideo"=w1198:string, "IFilterGraph2"=w1201:refnum<k24>, "Video"=w1195:T3, "Audio"=w1194:T3, "FrameGrabber?"=w1192:bool, "Preview?"=w1191:bool, "ICaptureGraphBuilder2"=w1186:refnum<k24>)
                    n513 = call "DirectShow - Media Control - Stop Preview.vi"("IFilterGraph2"=w1201, "Video"=w1195, "Audio"=w1194, "FrameGrabber?"=w1192) -> ("IFilterGraph2 dup"=w1196:refnum<k24>, "error out"=w1193:errorcluster)  [unwired: 10 in]
                    n514 = case shown="True" w1191 {
                      tunnel: w1200 -> [_ w1220]
                      tunnel: w1199 -> [_ w1219]
                      tunnel: w1198 -> [_ w1218]
                      tunnel: w1197 -> [_ w1217]
                      tunnel: w1196 -> [_ w1216]
                      tunnel: w1195 -> [_ w1215]
                      tunnel: w1194 -> [_ w1214]
                      tunnel: w1193 -> [w1205 w1213]
                      tunnel: w1192 -> [_ w1212]
                      tunnel: [DirectShow_-_Media_State."Stopped" ("MediaState") DirectShow_-_Media_State."Playing" ("MediaState")] -> w1190
                      tunnel: [-1 ("Timeout") 250 ("Timeout")] -> w1189
                      tunnel: [w1205 w1209] -> w1185
                      frame False {
                        w1206 = T4."Disabled and Grayed Out" ("Disabled")
                        n515 = property on="Run" class="Bool"("DisabledEnum"=w1206) -> ()  [unwired: 2 in, 2 out]
                        n516 = property on="Stop" class="Bool"("DisabledEnum"=w1206) -> ()  [unwired: 2 in, 2 out]
                        n517 = property on="Pause" class="Bool"("DisabledEnum"=w1206) -> ()  [unwired: 2 in, 2 out]
                      }
                      frame True {
                        n518 = case shown="False" w1220 {
                          tunnel: w1219 -> [_ w1229]
                          tunnel: [w1224 w1228] -> w1222
                          tunnel: [w1223 w1227] -> w1221
                          tunnel: w1218 -> [w1225 _]
                          frame False {
                            n519 = Scan From String(format string="%s %dx%d,%.2ffps,%dbit", input string=w1225) -> (output 2=w1224:i32, output 3=w1223:i32)  [unwired: 10 in, 3 out]
                          }
                          frame True {
                            n520 = property class="Pane"(reference=w1229) -> ("ContentBnds"=w1234:T8)  [unwired: 1 in, 2 out]
                            n521 = Unbundle(w1234) -> ("left"=w1230:i16, "top"=w1232:i16, "right"=w1231:i16, "bottom"=w1233:i16)
                            n522 = Subtract(x=w1231, y=w1230) -> (x-y=w1227:i16)
                            n523 = Subtract(x=w1233, y=w1232) -> (x-y=w1228:i16)
                          }
                        }
                        n524 = call "DirectShow - Media Control - Start Preview.vi"("IFilterGraph2"=w1216, "PictureBox"=w1217, "width"=w1222, "height"=w1221, "Video"=w1215, "Audio"=w1214, "FrameGrabber?"=w1212, "error in (no error)"=w1213) -> ("error out"=w1209:errorcluster)  [unwired: 6 in, 1 out]
                      }
                    }
                    n525 = call "DirectShow - Release Object.vi"("o"=w1186, "error in (no error)"=w1185) -> ("error out"=w1188:errorcluster)  [unwired: 13 in]
                    n526 = call "DirectShow - Create CaptureGraphBuilder.vi"("error in (no error)"=w1188) -> ("ICaptureGraphBuilder2"=w1187:refnum<k24>)  [unwired: 13 in, 1 out]
                    n527 = Bundle By Name(cluster=w1202, "Capture?"=FALSE, "Timeout"=w1189, "MediaState"=w1190, "ICaptureGraphBuilder2"=w1187) -> (w1204:T6)
                  }
                  frame True {
                    n528 = local read "Capture Folder"() -> (w1239:path)
                    n529 = call "Build File Name.vi"("Folder"=w1239, "Extension"="avi" ("pattern (all files)")) -> ("Path Out"=w1235:path, "File Path"=w1236:path, "Error"=w1237:errorcluster)  [unwired: 2 in, 1 out]
                    n530 = case shown="No Error" w1237 {
                      tunnel: [w1266 w1310] -> w1241
                      tunnel: w1240 -> [w1265 w1310]
                      tunnel: w1236 -> [w1243 _]
                      tunnel: w1235 -> [w1242 _]
                      frame No Error {
                        w1257 = T4."Enabled" ("Disabled")
                        n531 = local write "Capture Folder"(w1242) -> ()
                        n532 = Unbundle By Name(w1265) -> ("Pane"=w1253:refnum<vi>, "ScaleWindow?"=w1254:bool, "CurrentVideo"=w1255:string, "Preview"=w1249:refnum<k24>, "FrameGrabber?"=w1246:bool, "ICaptureGraphBuilder2"=w1267:refnum<k24>, "IFilterGraph2"=w1260:refnum<k24>, "Preview?"=w1250:bool, "Video"=w1245:T3, "Audio"=w1244:T3, "VideoC.Name"=w1263:string, "AudioC.Name"=w1262:string)
                        n533 = property on="Run" class="Bool"("DisabledEnum"=w1257) -> ()  [unwired: 2 in, 2 out]
                        n534 = property on="Stop" class="Bool"("DisabledEnum"=w1257) -> ()  [unwired: 2 in, 2 out]
                        n535 = property on="Pause" class="Bool"("DisabledEnum"=w1257) -> ()  [unwired: 2 in, 2 out]
                        n536 = case shown="True" w1254 {
                          tunnel: w1253 -> [_ w1304]
                          tunnel: w1255 -> [w1300 _]
                          tunnel: [w1299 w1303] -> w1248
                          tunnel: [w1298 w1302] -> w1247
                          frame False {
                            n537 = Scan From String(format string="%s %dx%d,%.2ffps,%dbit", input string=w1300) -> (output 2=w1299:i32, output 3=w1298:i32)  [unwired: 10 in, 3 out]
                          }
                          frame True {
                            n538 = property class="Pane"(reference=w1304) -> ("ContentBnds"=w1309:T8)  [unwired: 1 in, 2 out]
                            n539 = Unbundle(w1309) -> ("left"=w1305:i16, "top"=w1307:i16, "right"=w1306:i16, "bottom"=w1308:i16)
                            n540 = Subtract(x=w1306, y=w1305) -> (x-y=w1303:i16)
                            n541 = Subtract(x=w1308, y=w1307) -> (x-y=w1302:i16)
                          }
                        }
                        n542 = Unbundle By Name(w1245) -> ("Name"=w1259:string)
                        n543 = Unbundle By Name(w1244) -> ("Name"=w1258:string)
                        n544 = call "DirectShow - Media Control - Stop Preview.vi"("IFilterGraph2"=w1260, "Video"=w1245, "Audio"=w1244, "FrameGrabber?"=w1246) -> ("IFilterGraph2 dup"=w1252:refnum<k24>, "error out"=w1251:errorcluster)  [unwired: 10 in]
                        n545 = case shown="True" w1250 {
                          tunnel: w1267 -> [w1278 w1297]
                          tunnel: w1263 -> [w1277 w1296]
                          tunnel: w1262 -> [w1276 w1295]
                          tunnel: w1259 -> [w1275 w1282]
                          tunnel: w1258 -> [w1274 w1281]
                          tunnel: w1243 -> [w1273 w1289]
                          tunnel: w1252 -> [w1272 w1285]
                          tunnel: w1251 -> [w1271 w1291]
                          tunnel: w1249 -> [_ w1284]
                          tunnel: w1248 -> [_ w1288]
                          tunnel: w1247 -> [_ w1287]
                          tunnel: w1246 -> [_ w1283]
                          frame False {
                            n546 = call "DirectShow - Configure Capture.vi"("IFilterGraph2"=w1272, "Path"=w1273, "ICaptureGraphBuilder2"=w1278, "Video"=w1275, "Audio"=w1274, "error in (no error)"=w1271, "VideoCompressor"=w1277, "AudioCompressor"=w1276) -> ("IFilterGraph2 2"=w1268:refnum<k24>, "error out"=w1270:errorcluster)  [unwired: 6 in]
                            n547 = call "DirectShow - Media Control - StartStopPause.vi"("IFilterGraph2"=w1268, "Mode"=DirectShow_-_Media_Mode."Run", "error in (no error)"=w1270) -> ()  [unwired: 11 in, 2 out]
                          }
                          frame True {
                            n548 = call "DirectShow - Init Capture Preview.vi"("IFilterGraph2"=w1285, "PictureBox"=w1284, "width"=w1288, "height"=w1287, "Video"=w1282, "Audio"=w1281, "FrameGrabber?"=w1283, "error in (no error)"=w1291) -> ("IFilterGraph2 dup"=w1286:refnum<k24>, "VideoSource"=w1280:refnum<k24>, "AudioSource"=w1279:refnum<k24>, "error out"=w1290:errorcluster)  [unwired: 4 in]
                            n549 = call "DirectShow - Configure Capture plus Preview.vi"("IFilterGraph2"=w1286, "Path"=w1289, "ICaptureGraphBuilder2"=w1297, "Video"=w1280, "Audio"=w1279, "error in (no error)"=w1290, "VideoCompressor"=w1296, "AudioCompressor"=w1295) -> ("IFilterGraph2 dup"=w1293:refnum<k24>, "error out"=w1292:errorcluster)  [unwired: 6 in]
                            n550 = call "DirectShow - Media Control - StartStopPause.vi"("IFilterGraph2"=w1293, "Mode"=DirectShow_-_Media_Mode."Run", "error in (no error)"=w1292) -> ()  [unwired: 11 in, 2 out]
                          }
                        }
                        n551 = Bundle By Name(cluster=w1265, "Capture?"=TRUE, "Timeout"=250, "MediaState"=DirectShow_-_Media_State."Recording") -> (w1266:T6)
                      }
                      frame Error {
                        n552 = call "Display Message to User"() -> ()  [unwired: 10 in, 2 out]
                      }
                    }
                  }
                }
              }
              event "Summary", "SnapSummary": Shortcut Menu Selection (User) {
                n553 = event-data() -> ("CtlRef"=w1321:refnum<vi>, "ItemPath"=w1317:string)  [unwired: 1 in]
                n554 = Unbundle By Name(w1318) -> ("FrameGrab"=w1312:refnum<k24>, "WindowSnap"=w1311:refnum<k24>)
                n555 = property class="Str"(reference=w1321) -> (reference out=w1319:refnum<vi>, error out=w1320:errorcluster, "Label.Text"=w1316:string)  [unwired: 1 in]
                n556 = Close Reference(reference=w1319, error in (no error)=w1320) -> ()  [unwired: 1 out]
                n557 = Equal?(x=w1316, y="Summary") -> (x = y?=w1314:bool)
                n558 = Select(t=w1312, s=w1314, f=w1311) -> (s? t:f=w1313:refnum<k24>)
                n559 = case shown="\"Save as BMP\"" w1317 {
                  tunnel: w1313 -> [_ w1328 w1351]
                  frame "False", Default {
                  }
                  frame "Save as BMP" {
                    n560 = property class="PictureBox"(reference=w1328) -> ("Image"=w1322:refnum<k24>)  [unwired: 1 in, 2 out]
                    n561 = call "File Dialog"("prompt"="Save as BMP...", "pattern (all files)"="*.bmp", "pattern label"="Bitmap Files") -> ("selected path"=w1323:path, "error out"=w1324:errorcluster)  [unwired: 9 in, 2 out]
                    n562 = case shown="No Error" w1324 {
                      tunnel: w1323 -> [w1340 _]
                      tunnel: w1322 -> [w1342 _]
                      frame No Error {
                        w1334 = refnum<k24> refnum  # ImageFormat
                        n563 = constructor class="Bitmap"("original"=w1342) -> (reference out=w1341:refnum<k24>, error out=w1332:errorcluster)  [unwired: 3 in, 2 out]
                        n564 = Path To String(path=w1340) -> (string=w1339:string)
                        n565 = property class="ImageFormat"(reference=w1334, error in=w1332) -> (reference out=w1330:refnum<k24>, error out=w1331:errorcluster, "Bmp"=w1333:refnum<k24>)
                        n566 = invoke class="Bitmap" method="Save"(reference=w1341, error in=w1331, "filename"=w1339, "format"=w1333) -> (reference out=w1338:refnum<k24>, error out=w1337:errorcluster)  [unwired: 1 in, 3 out]
                        n567 = invoke class="Bitmap" method="Dispose"(reference=w1338, error in=w1337) -> (reference out=w1335:refnum<k24>, error out=w1336:errorcluster)  [unwired: 1 in, 1 out]
                        n568 = Close Reference(reference=w1335, error in (no error)=w1336) -> (error out=w1329:errorcluster)
                        n569 = Close Reference(reference=w1330, error in (no error)=w1329) -> ()  [unwired: 1 out]
                      }
                      frame Error {
                      }
                    }
                  }
                  frame "Copy as LabVIEW Image" {
                    n570 = property class="PictureBox"(reference=w1351) -> ("Image"=w1350:refnum<k24>)  [unwired: 1 in, 2 out]
                    n571 = constructor class="Bitmap"("original"=w1350) -> (reference out=w1349:refnum<k24>, error out=w1348:errorcluster)  [unwired: 3 in, 2 out]
                    n572 = call "DirectShow - Bitmap to LabVIEW Image.vi"("Bitmap"=w1349, "error in (no error)"=w1348) -> ("Bitmap dup"=w1347:refnum<k24>, "LV_Image"=w1343:T11, "error out"=w1346:errorcluster)  [unwired: 10 in, 1 out]
                    n573 = call "DirectShow - Show LabVIEW Image.vi"("image data"=w1343) -> ()  [unwired: 15 in]
                    n574 = invoke class="Bitmap" method="Dispose"(reference=w1347, error in=w1346) -> (reference out=w1344:refnum<k24>, error out=w1345:errorcluster)  [unwired: 1 in, 1 out]
                    n575 = Close Reference(reference=w1344, error in (no error)=w1345) -> ()  [unwired: 1 out]
                  }
                }
              }
            }
          }
        }
      }
    }
    frame #2 {
      w1352 = ""
      n576 = local write "Capture Folder"(path "") -> ()
      n577 = local write "Source Name"(w1352) -> ()
      n578 = local write "AutorunText"(w1352) -> ()
      n579 = local write "AutocloseText"(w1352) -> ()
      n580 = property class="App"() -> ("App.Kind"=w1355:T12)  [unwired: 2 in, 2 out]
      n581 = control-ref of="Dieses VI"() -> (w1354:refnum<vi>)
      n582 = case shown="\"Development System\"" w1355 {
        tunnel: w1354 -> [w1356 w1358]
        frame "invalid app kind", Default {
          n583 = invoke on="Invoke Node" class="VI" method="FP.Close"(reference=w1356) -> ()  [unwired: 2 in, 3 out]
        }
        frame "Development System" {
          n584 = case shown="False" "Autoclose" {
            tunnel: w1358 -> [_ w1359]
            frame False {
            }
            frame True {
              n585 = invoke on="Invoke Node" class="VI" method="FP.Close"(reference=w1359) -> ()  [unwired: 2 in, 3 out]
            }
          }
        }
      }
    }
  }
